vi "Text control 2 v6.2.vi"() -> ()   [LabVIEW 2016]
panel:
  in  "Tab Control":enum32{"Main", "Other parameters"}(tab)
  out "Line running":i32
  out "Total lines":i32
  out "Path":path=path "C:/users/rlp38/09Apr2009LTtesting/test2.txt"
  out "I vs Vg":cluster{"Y data in":dbl[], "X data in":dbl[]}[](graph)
  out "Is max":dbl format="%.2e"
  out "Id max":dbl format="%.2e"
  out "Ig max":dbl format="%.2e"
  out "Imax vs time":cluster{"Y data in":dbl[], "X data in":dbl[]}[](graph)
  out "Imin vs time":cluster{"Y data in":dbl[], "X data in":dbl[]}[](graph)
  out "I vs Vd":cluster{"Y data in":dbl[], "X data in":dbl[]}[](graph)
  in  "Script":string="#pulsedstressV d 0.03 20 0 0.5 0.0827 5\n#\n#itime m\n#gaterangemode a\n#drainrangemode a\n#pulsed on 0.05 0 0.02\n#transfer d -10 40 1 5 40 35\n#transfer d -10 40 1 5 40 35\n#transfer d -10 40 1 5 40 35\n#output d 0 40 20 0 40 1\n#\n#\n#sample 1 0.008 221 6 0.003\n#samplei 400e-6 200 6 0.002 0.1\n#vsu2pulse -10 4\n#\n#stressV 0.016 0.03 2e-4 0.1e-3 11\n#stressI 220e-7 0.08 15\n#transfer s -1 1 0.5 -0.005 0.005 0.005\n#output s 0 0 0 -0.008 0.008 0.002"
  out "Command running:":string
  out "Serial port data":string
  out "Elapsed Time":dbl caption="Elapsed Time (s)"
  in  "Time Units":u16(ring)=1 items=["Seconds", "Minutes", "Hours"]
  in  "Time Offset":dbl caption="Set Start Time (s)"
  in  "Reset":bool
  in  "Auto Reset":bool
  in  "integration time":u32(slide) max=2 step=1 scale=0.0..2.0
  out "Is on":dbl format="%.2e"
  out "Id on":dbl format="%.2e"
  out "Ig on":dbl format="%.2e"
  out "Ion vs time":cluster{"Y data in":dbl[], "X data in":dbl[]}[](graph)
  out "Ioff vs time":cluster{"Y data in":dbl[], "X data in":dbl[]}[](graph)
  out "Ig min":dbl format="%.2e"
  out "Id min":dbl format="%.2e"
  out "Is min":dbl format="%.2e"
  out "Is off":dbl format="%.2e"
  out "Id off":dbl format="%.2e"
  out "Ig off":dbl format="%.2e"
  in  "Integration time (long)":dbl=0.32 min=0.04 max=2.0 step=0.02 format="%.2f"
  in  "Integration time (short)":dbl=0.0019 min=8e-05 max=0.0019 step=8e-05 format="%^.0e"
  in  "Drain: Compliance":dbl=0.001 format="%.8f"
  in  "Gate: Compliance":dbl=0.001 format="%.8f"
  in  "Interrupt scan":bool
  in  "Standby":T1
  in  "Full Reset":bool
  in  "SMU4":cluster{"on/off":bool, "Voltage":dbl} {"Voltage" min=-100.0 max=100.0 format="%.2f"}
  in  "Interrupt program":bool
  in  "Gate Range\nmode":u16(ring) items=["Auto", "Limited", "Fixed"]
  in  "Gate Range":u8(slide)=6 max=11 scale=0.0..11.0
  in  "Source/Drain\nRange mode":u16(ring) items=["Auto", "Limited", "Fixed"]
  in  "Source/Drain Range":u8(slide)=6 max=11 scale=0.0..11.0
  in  "Panel Controls":T2={"Emergency Stop"=refnum, "TransGraph Max"=1e-05, "Text/Graph (text=false)"=TRUE} {"TransGraph Max" format="%.2e"}
  in  "Panel Controls 2":T3={"Emergency Stop"=refnum, "TransGraph Max"=1e-05, "Text/Graph (text=false)"=TRUE, "TransGraph Min"=1e-11} {"TransGraph Min" format="%.2e"; "TransGraph Max" format="%.2e"}
  out "error out":errorcluster
  in  "Delay before read (ms)":u32=1000
  in  "byte count":u32=64
  in  "Serial End Mode for Reads":u16(ring)=2 items=["None", "LastBit", "TermChar"]
  in  "Timeout (ms)":u32=10000
  in  "Enable Termination\nChar (T)":bool=TRUE
  in  "Termination char\n(0xA = '\\n' = LF)\n(0xD = '\\r' = CR)":u8=13 format="%.0x"
  in  "flow control":u16(ring) items=["None"=0, "XON/XOFF"=1, "RTS/CTS"=2, "DTR/DSR"=4]
  in  "stop bits":u16(ring)=10 items=["1.0"=10, "1.5"=15, "2.0"=20]
  in  "parity":u16(ring) items=["None", "Odd", "Even", "Mark", "Space"]
  in  "data bits":u16=8 min=5 max=8 step=1
  in  "VISA resource name":refnum<visa-resource-name>="COM6"
  in  "baud rate":u32=9600
  out "Timings Indicator":T4
  in  "Timings (overwritten by the Front Panel)":T5={"integration time"=0, "Short/Long integration time"=0.00064, "hold time (sec)"=0.0, "delay time (sec)"=0.0, "Step Time (0 disables)"=0.0, "sweep method"=0, "Pulse period"=0.005, "Base voltage"=0.0, "Pulse width"=0.0005} {"Pulse width" min=0.0005 max=0.1 step=0.0001 format="%.4f"; "Base voltage" format="%^.4e"; "Pulse period" min=0.005 max=1.0 step=0.0001 format="%.4f"; "sweep method" items=["Continuous", "Pulsed"]; "Step Time (0 disables)" format="%.2f"; "delay time (sec)" format="%.4f"; "hold time (sec)" format="%.4f"; "Short/Long integration time" format="%^.0e"; "integration time" scale=0.0..2.0}
  in  "Gate":T6={"Gate Start"=0.0, "Gate Stop"=2.0, "Gate Step (linear only)"=1.0, "Gate Compliance"=0.0001, "Gate PComp"=0.0, "Range mode"=0, "Range"=6} {"Range" max=11 scale=0.0..11.0; "Range mode" items=["Auto", "Limited", "Fixed"]; "Gate PComp" format="%^.2e"; "Gate Compliance" format="%^.2e"; "Gate Step (linear only)" format="%^.4e"; "Gate Stop" format="%^.4e"; "Gate Start" format="%^.4e"}
  in  "Drain 2":T7={"Drain Start"=0.0, "Drain Stop"=2.0, "Drain Compliance"=0.0001, "Drain Step"=1.0, "Drain PComp"=0.0, "Range mode"=0, "Range"=6} {"Range" max=11 scale=0.0..11.0; "Range mode" items=["Auto", "Limited", "Fixed"]; "Drain PComp" format="%^.2e"; "Drain Step" format="%^.4e"; "Drain Compliance" format="%^.2e"; "Drain Stop" format="%^.4e"; "Drain Start" format="%^.4e"}
  # "Time"
  # "Syntax:\nitime [s|m|l] time(sec): [s|m|l] determines the integration time setting (small|medium|long) and time sets the value.\nNOTE: The value of the integration time has to be within the range allowed by its category (s|m|l), otherwise, the closest value will be used. (e.g. if the category is set to short but the time value is very long, the actual value used will be the maximum short integration time.\nIntegration times:\n    Short: Default: 640 us. Range: 8E-5 - 1.92E-3 seconds.\n    Medium: Fixed at 1 NPL cycle (0.02 seconds).\n    Long: Default: 16 NPL cycles (0.32 seconds). Range: 2-100 NPL cycles (0.04 seconds - 2 seconds).\ngaterangemode [a|l|f]\ndrainrangemode [a|l|f]\npulsed [on|off] PulsePeriod(sec) PulseBaseVoltage PulseONWidth(sec)\nstandby [on l off]\nwait NumMilliseconds\nwait-min NumMinutes\n# texthere = comment\ntransfer [s|d] VgStart VgStop VgStep VdStart VdStop VdStep\noutput [s|d] VgStart VgStop VgStep VdStart VdStop VdStep\nsample Vg Vd NumSamples Time(s) SampleInterval(s)\nsamplei Idg NumSamples Time(s) SampleInterval(s) VDGcompliance\n100 samples is approximately 13 seconds with medium integration\n# if in doubt use SampleInterval(s) = 0.004\nstressV VG VD IGcompliance IDcompliance Duration(sec)\nstressI IDG VDGcompliance Duration(sec)\nvsu2pulse Bias Duration(s)\npulsedstressV [s|d] VEstop VgON VgOFF Period(s) PulseONwidth(s) Vd\nsample-fpp Vg Vd NumSamples Time\nresample-fpp Vg Vd\ntransfer-fpp [s|d] VgStart VgStop VgStep VdStart VdStop VdStep\noutput-fpp [s|d] VgStart VgStop VgStep VdStart VdStop VdStep\nserial SerialPortCommand"
  # "1\n2\n3\n4\n5\n6\n7\n8\n9\n10\n11\n12\n13\n14\n15\n16\n17\n18\n19\n20"
  # "Serial port settings"
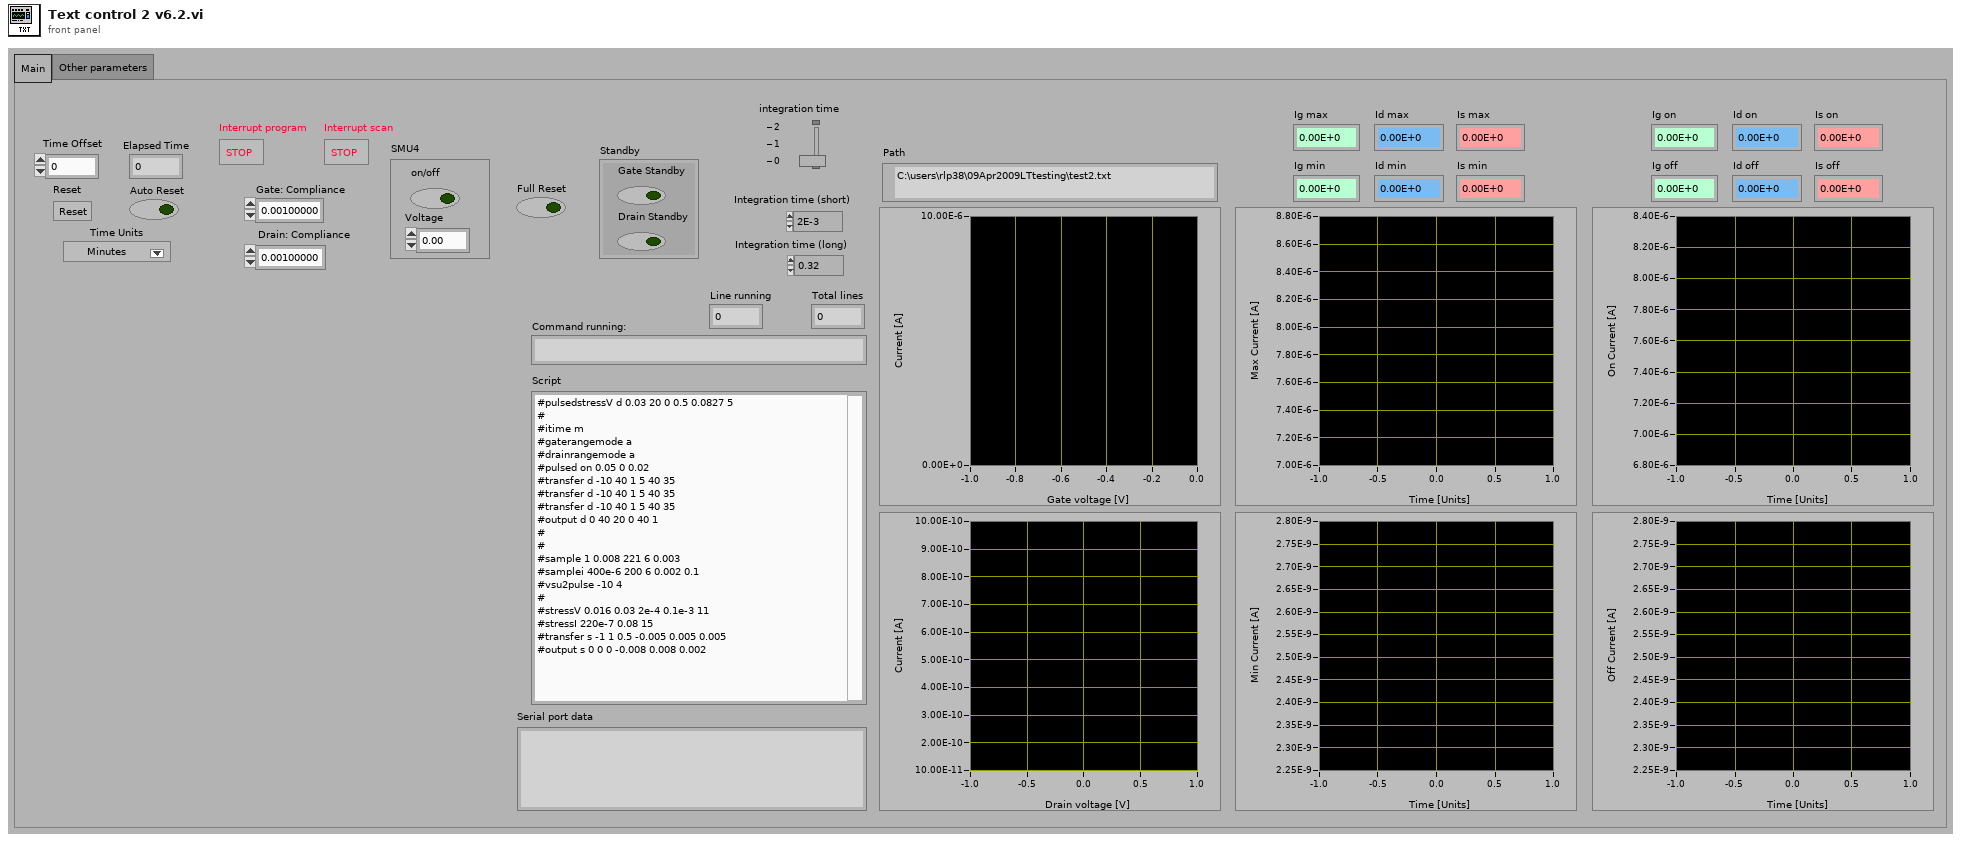
[diagram p1: front panel]
types:
  T1 = cluster{"Gate Standby":bool, "Drain Standby":bool}
  T2 = cluster{"Emergency Stop":refnum<vi>, "TransGraph Max":dbl, "Text/Graph (text=false)":bool}
  T3 = cluster{"Emergency Stop":refnum<vi>, "TransGraph Max":dbl, "Text/Graph (text=false)":bool, "TransGraph Min":dbl}
  T4 = cluster{"integration time (0:s, 1:m, 2:l)":u32, "Short/Long integration time":dbl, "hold time (sec)":dbl, "delay time (sec)":dbl, "Step Time (0 disables)":dbl, "sweep method":u16, "Pulse period":dbl, "Base voltage":dbl, "Pulse width":dbl}
  T5 = cluster{"integration time":u32, "Short/Long integration time":dbl, "hold time (sec)":dbl, "delay time (sec)":dbl, "Step Time (0 disables)":dbl, "sweep method":u16, "Pulse period":dbl, "Base voltage":dbl, "Pulse width":dbl}
  T6 = cluster{"Gate Start":dbl, "Gate Stop":dbl, "Gate Step (linear only)":dbl, "Gate Compliance":dbl, "Gate PComp":dbl, "Range mode":u16, "Range":u8}
  T7 = cluster{"Drain Start":dbl, "Drain Stop":dbl, "Drain Compliance":dbl, "Drain Step":dbl, "Drain PComp":dbl, "Range mode":u16, "Range":u8}
  T8 = enum16{"open", "replace", "create", "open or create", "replace or create", "replace or create with confirmation"}
  T9 = cluster{"V2 Start":dbl, "V2 Step":dbl, "Number of points":i32}
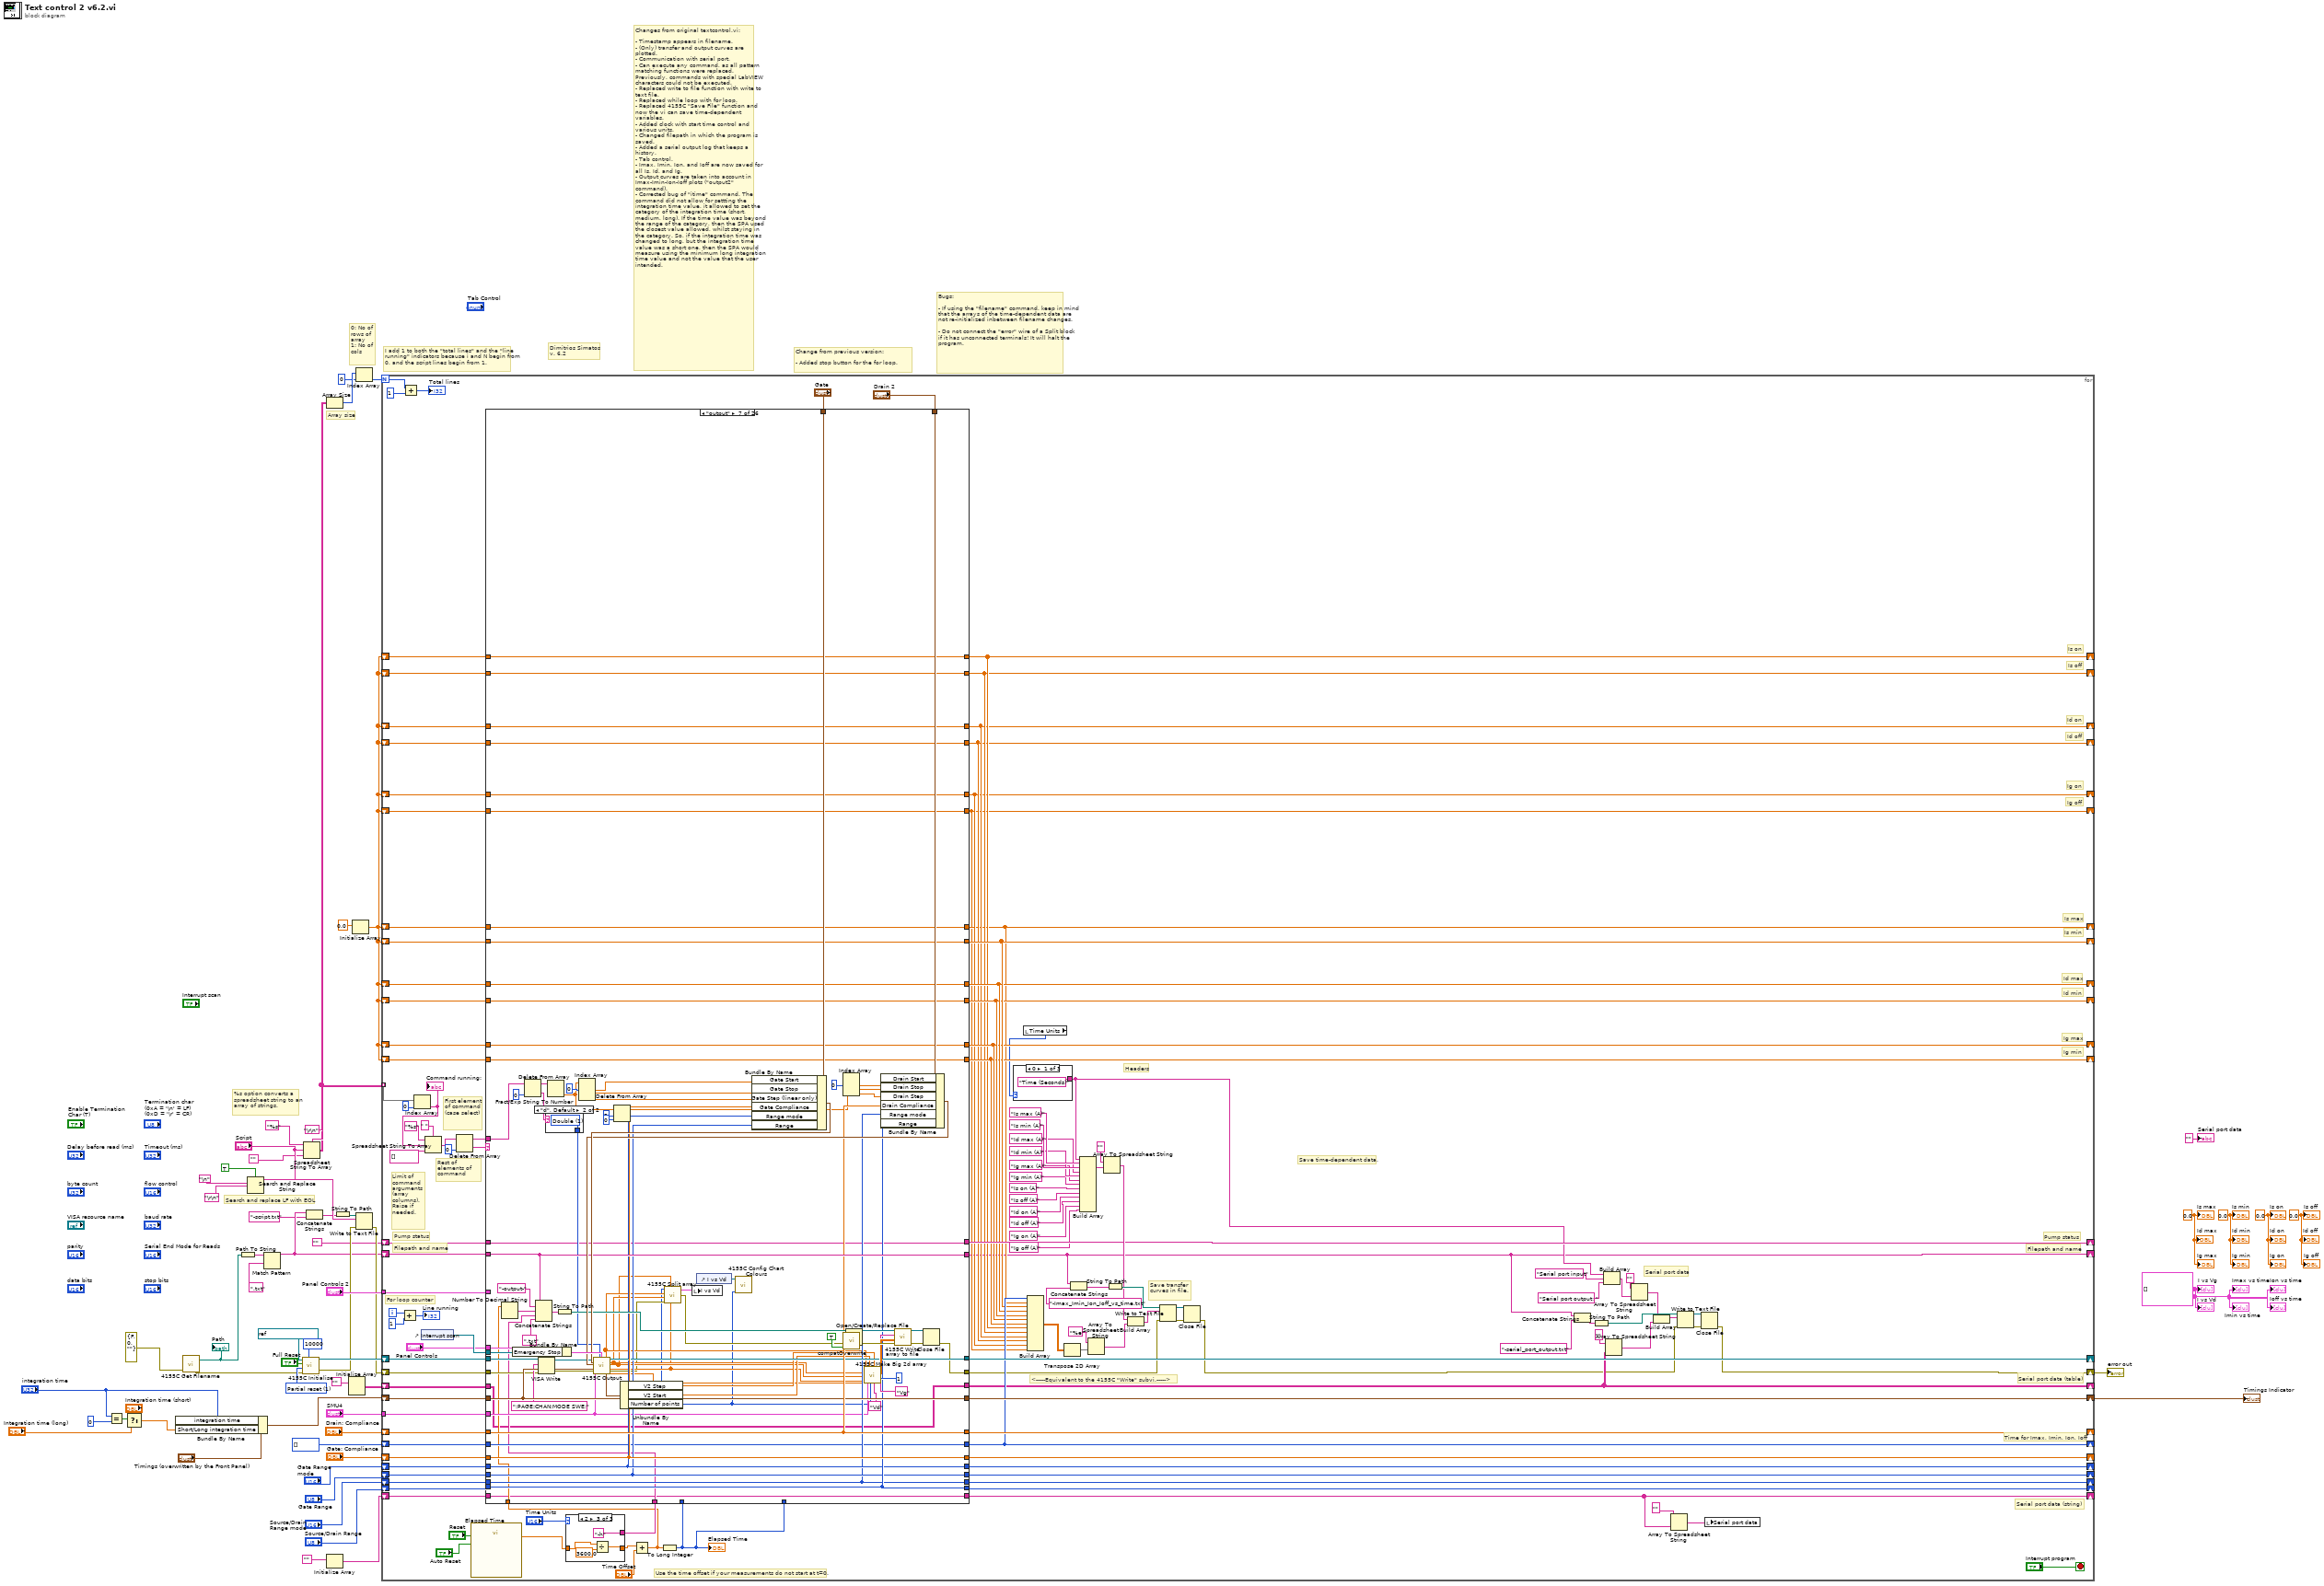
[diagram p0: block diagram]
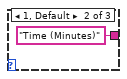
[diagram p2: hidden frame]
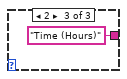
[diagram p3: hidden frame]
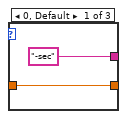
[diagram p4: hidden frame]
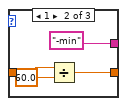
[diagram p5: hidden frame]
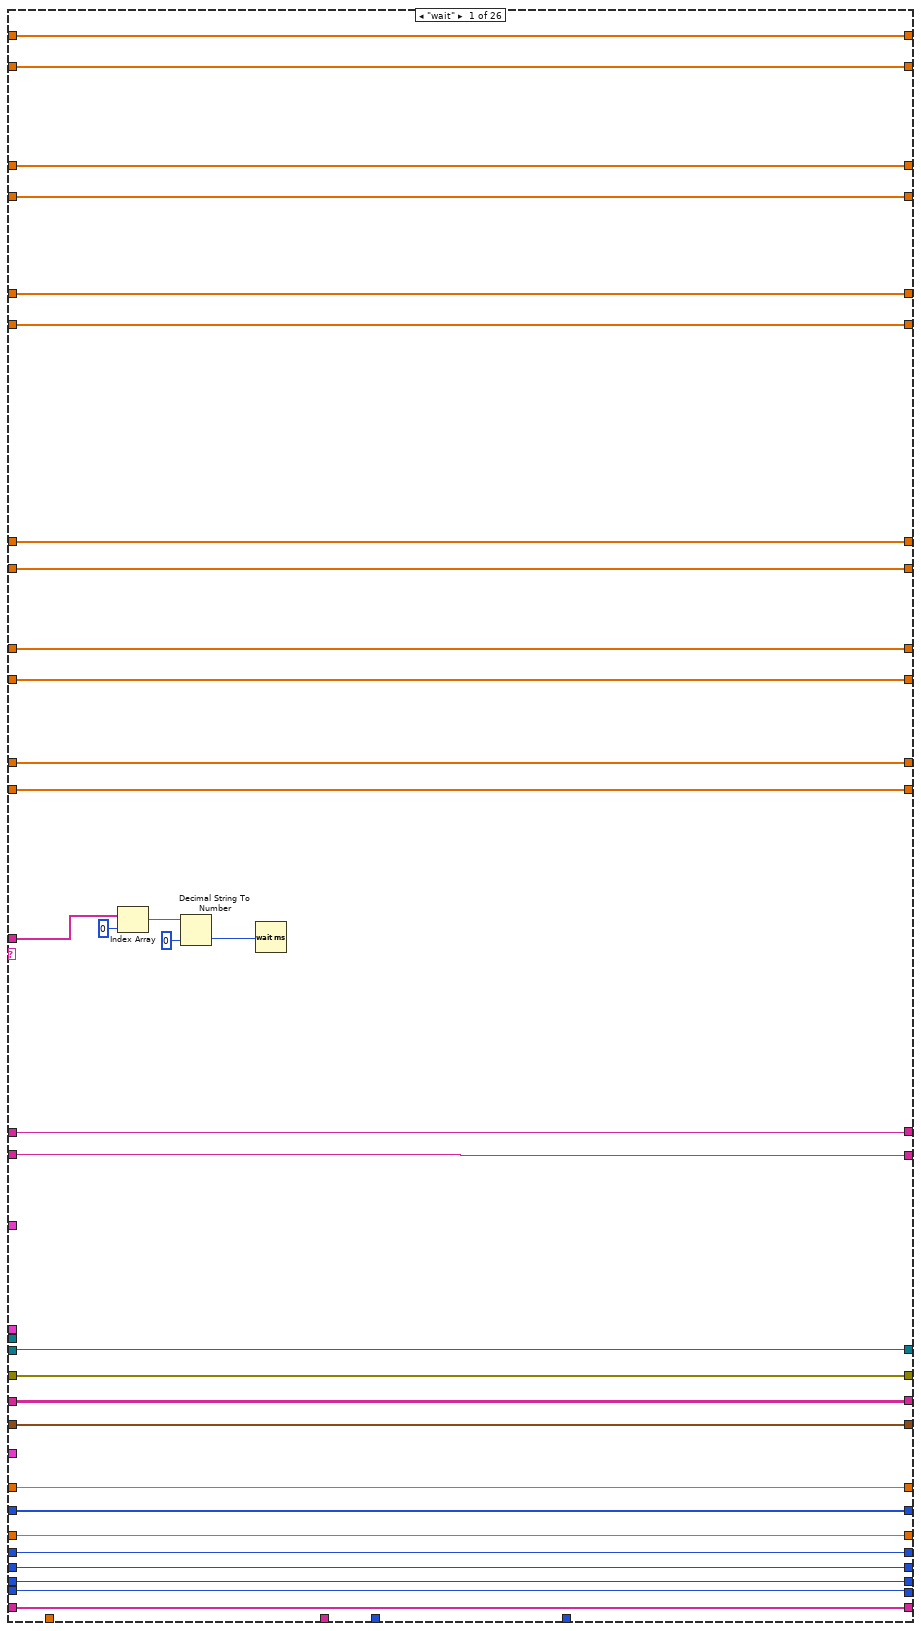
[diagram p6: hidden frame]
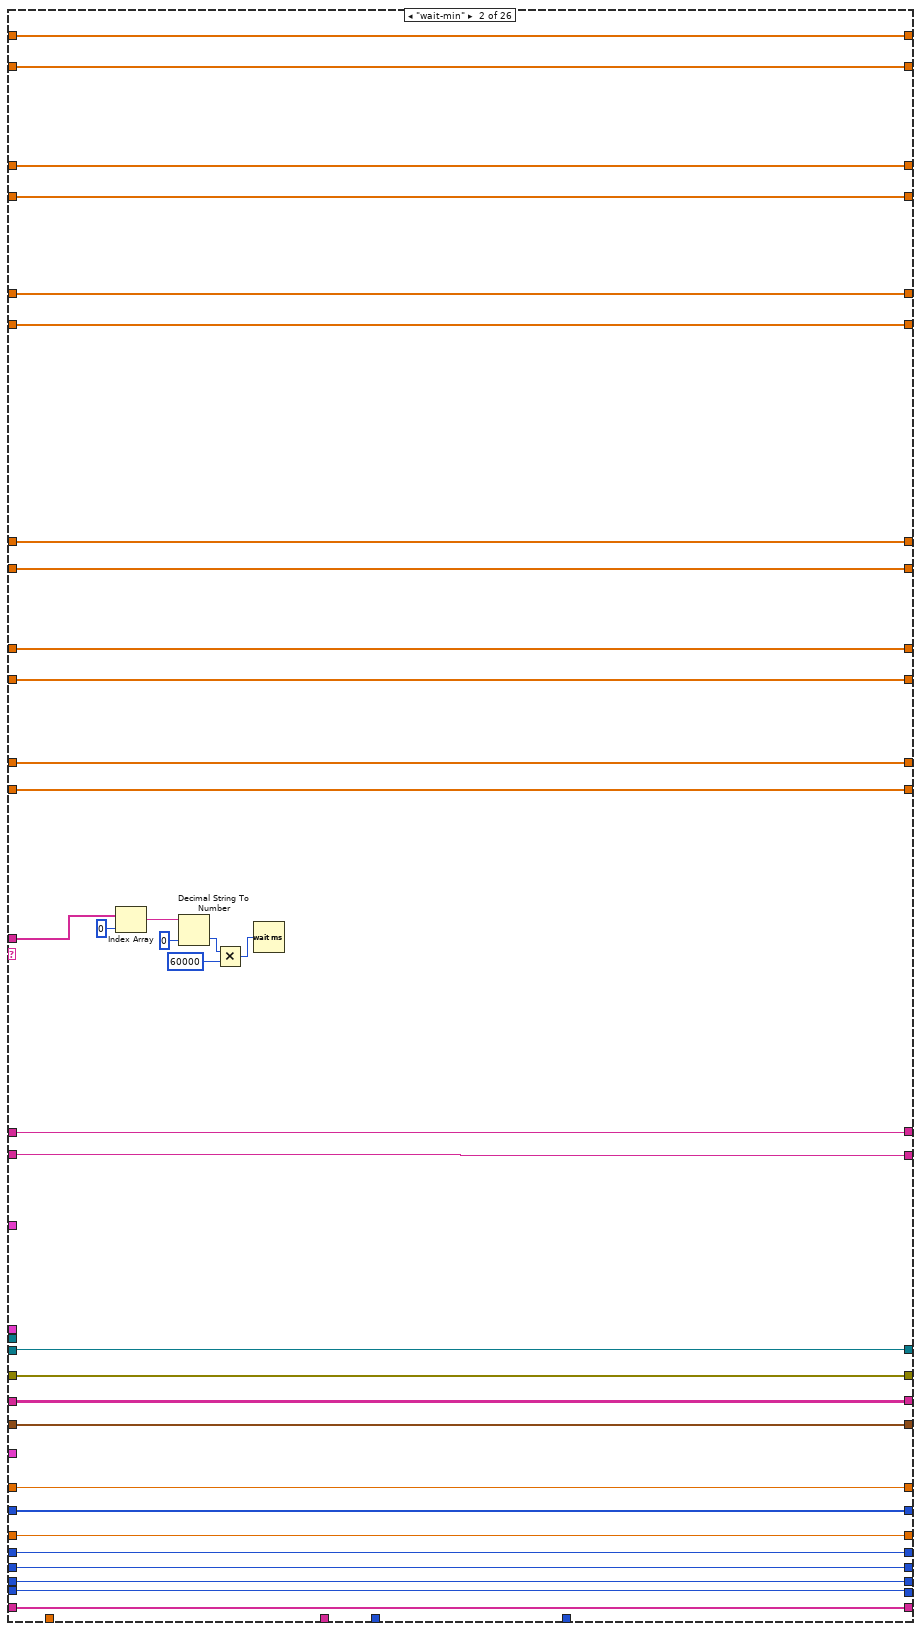
[diagram p7: hidden frame]
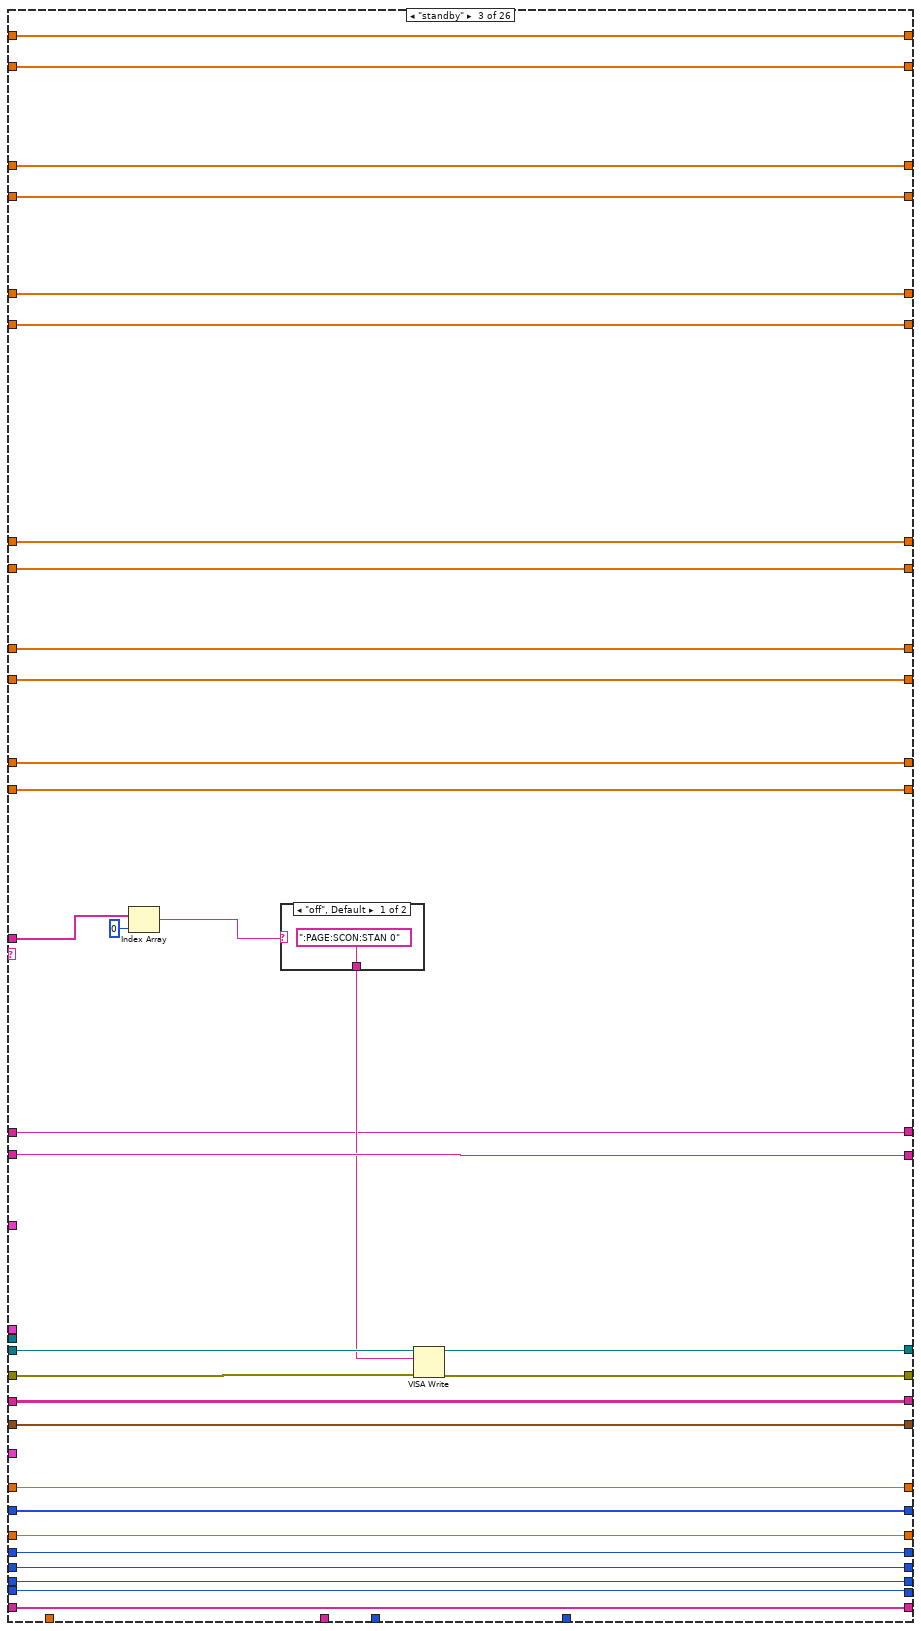
[diagram p8: hidden frame]
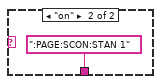
[diagram p9: hidden frame]
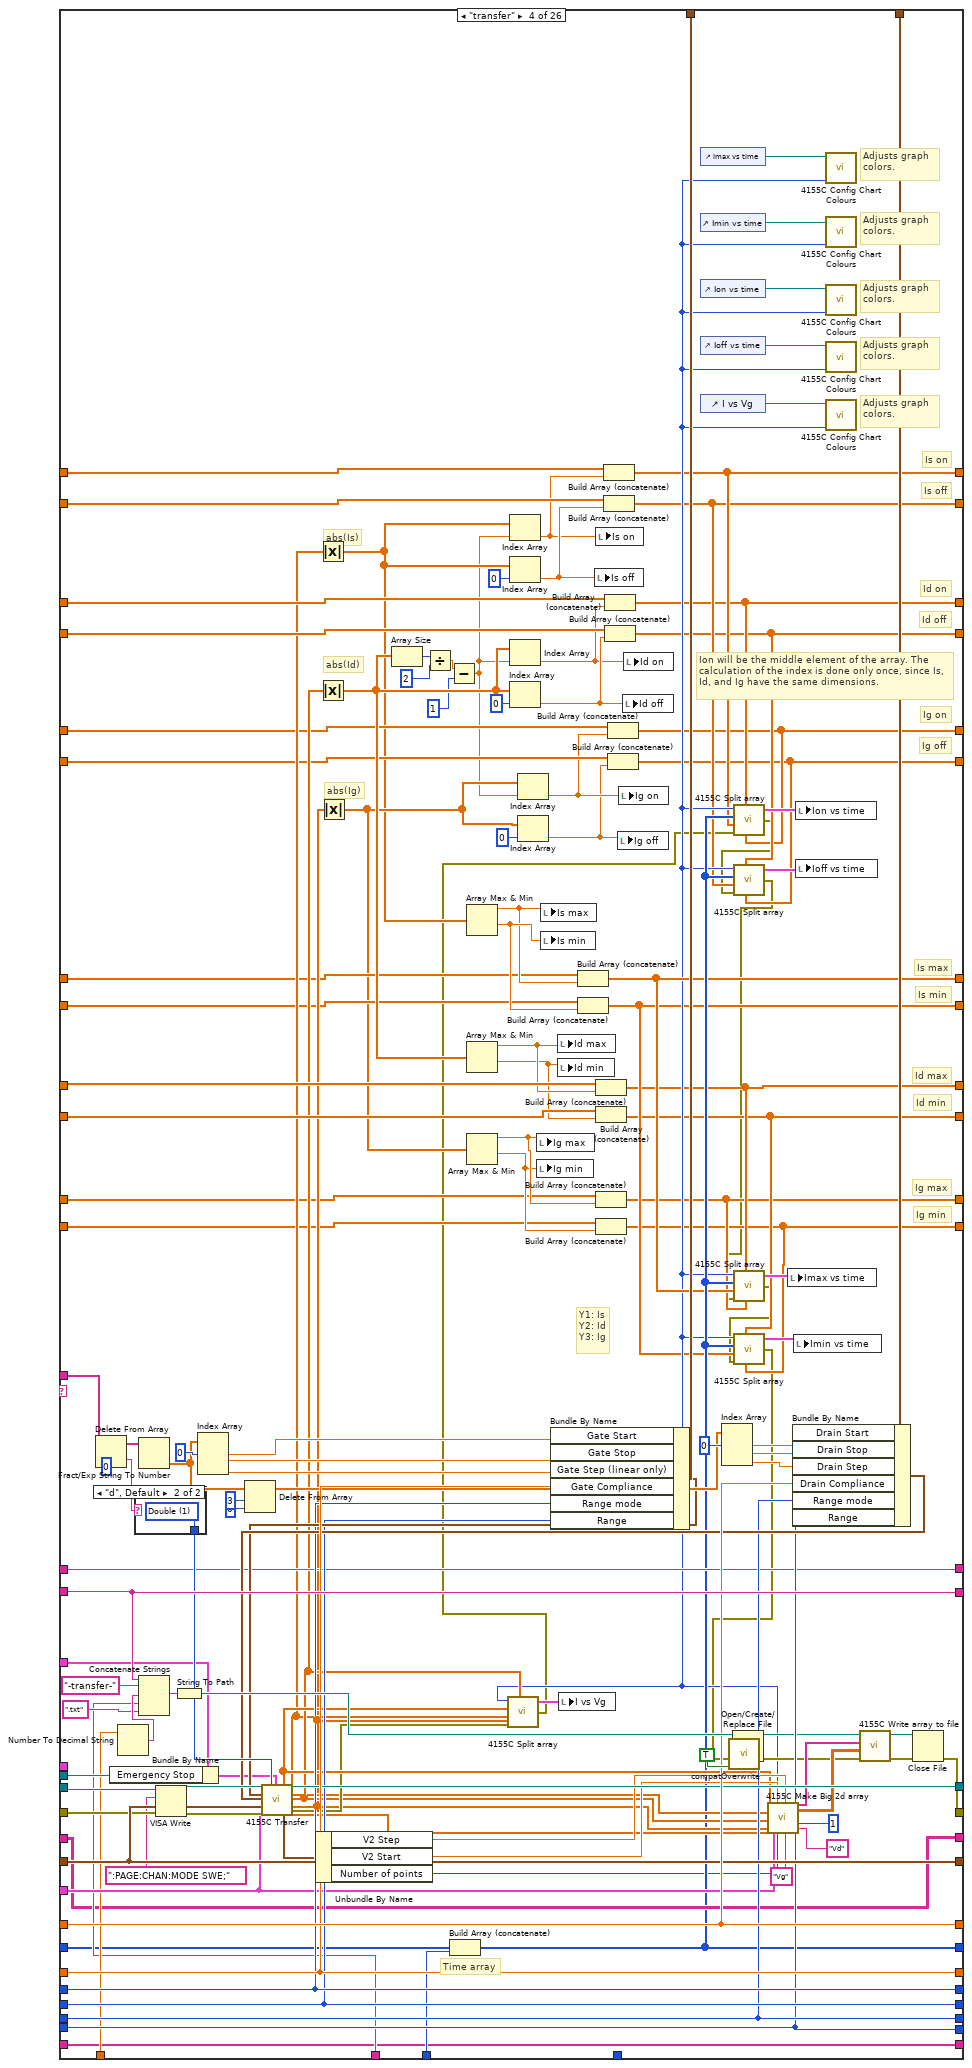
[diagram p10: hidden frame]
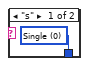
[diagram p11: hidden frame]
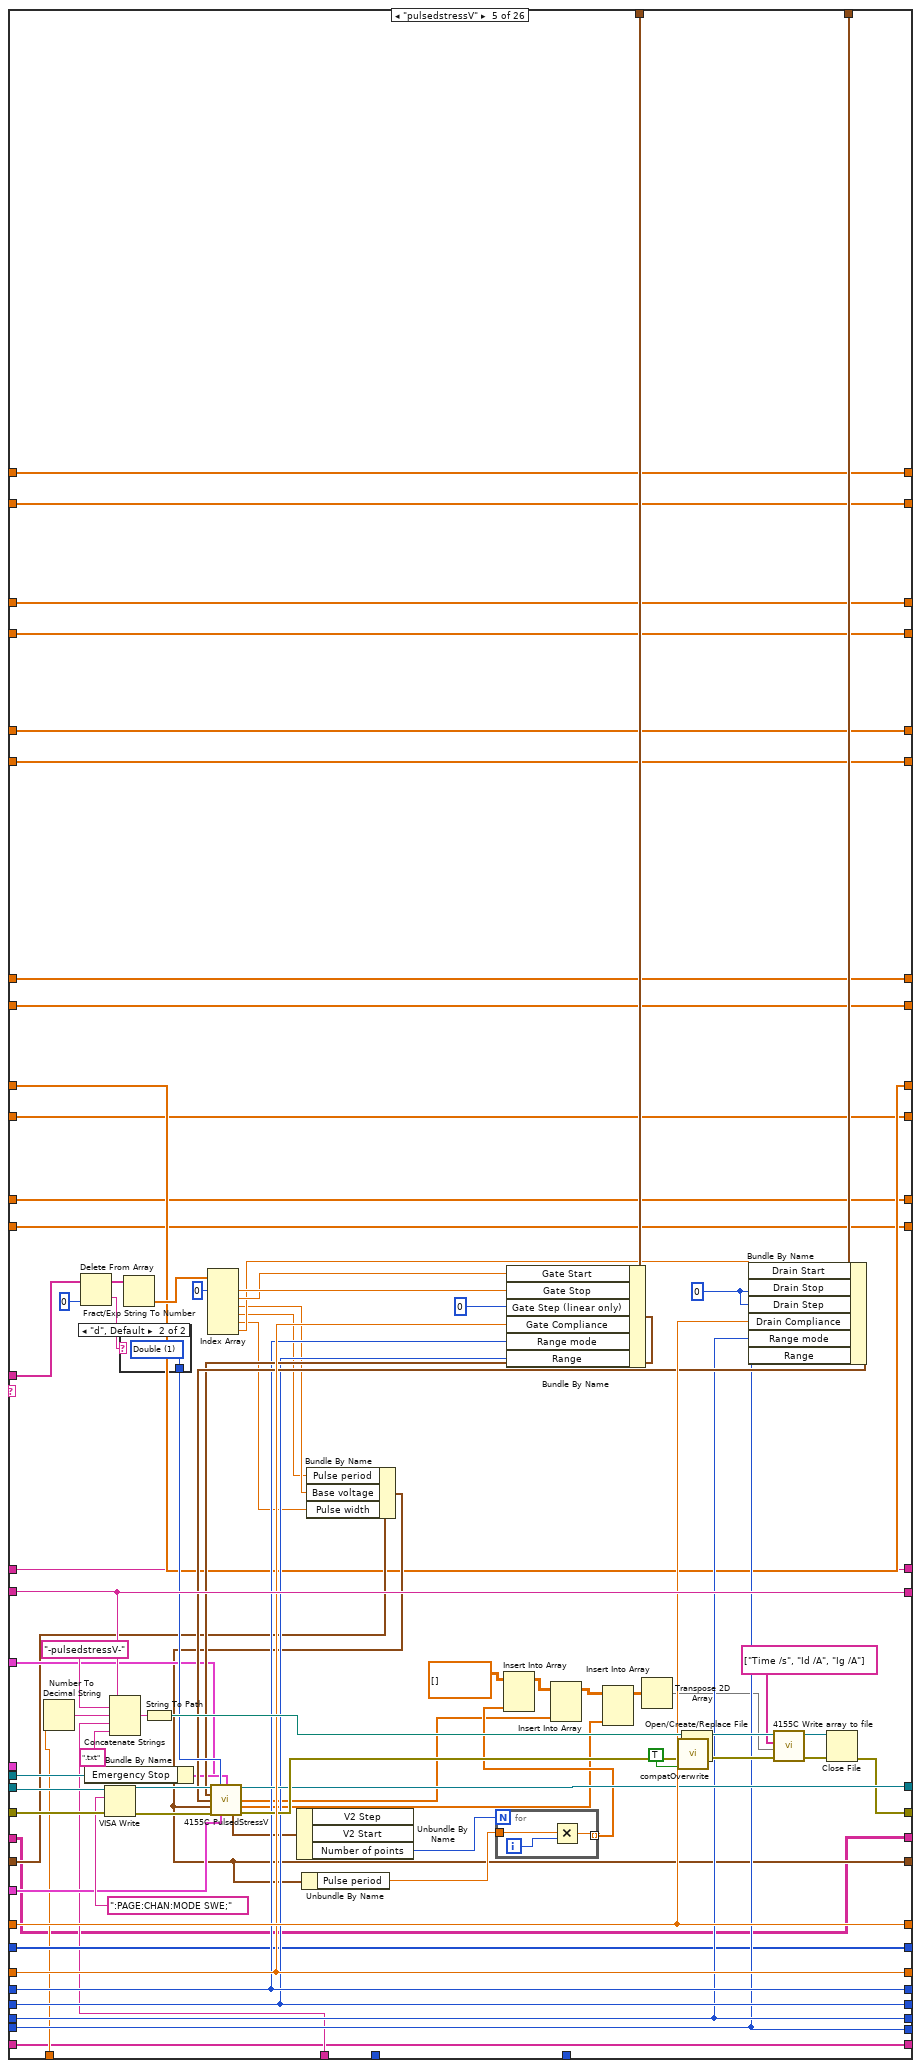
[diagram p12: hidden frame]
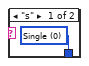
[diagram p13: hidden frame]
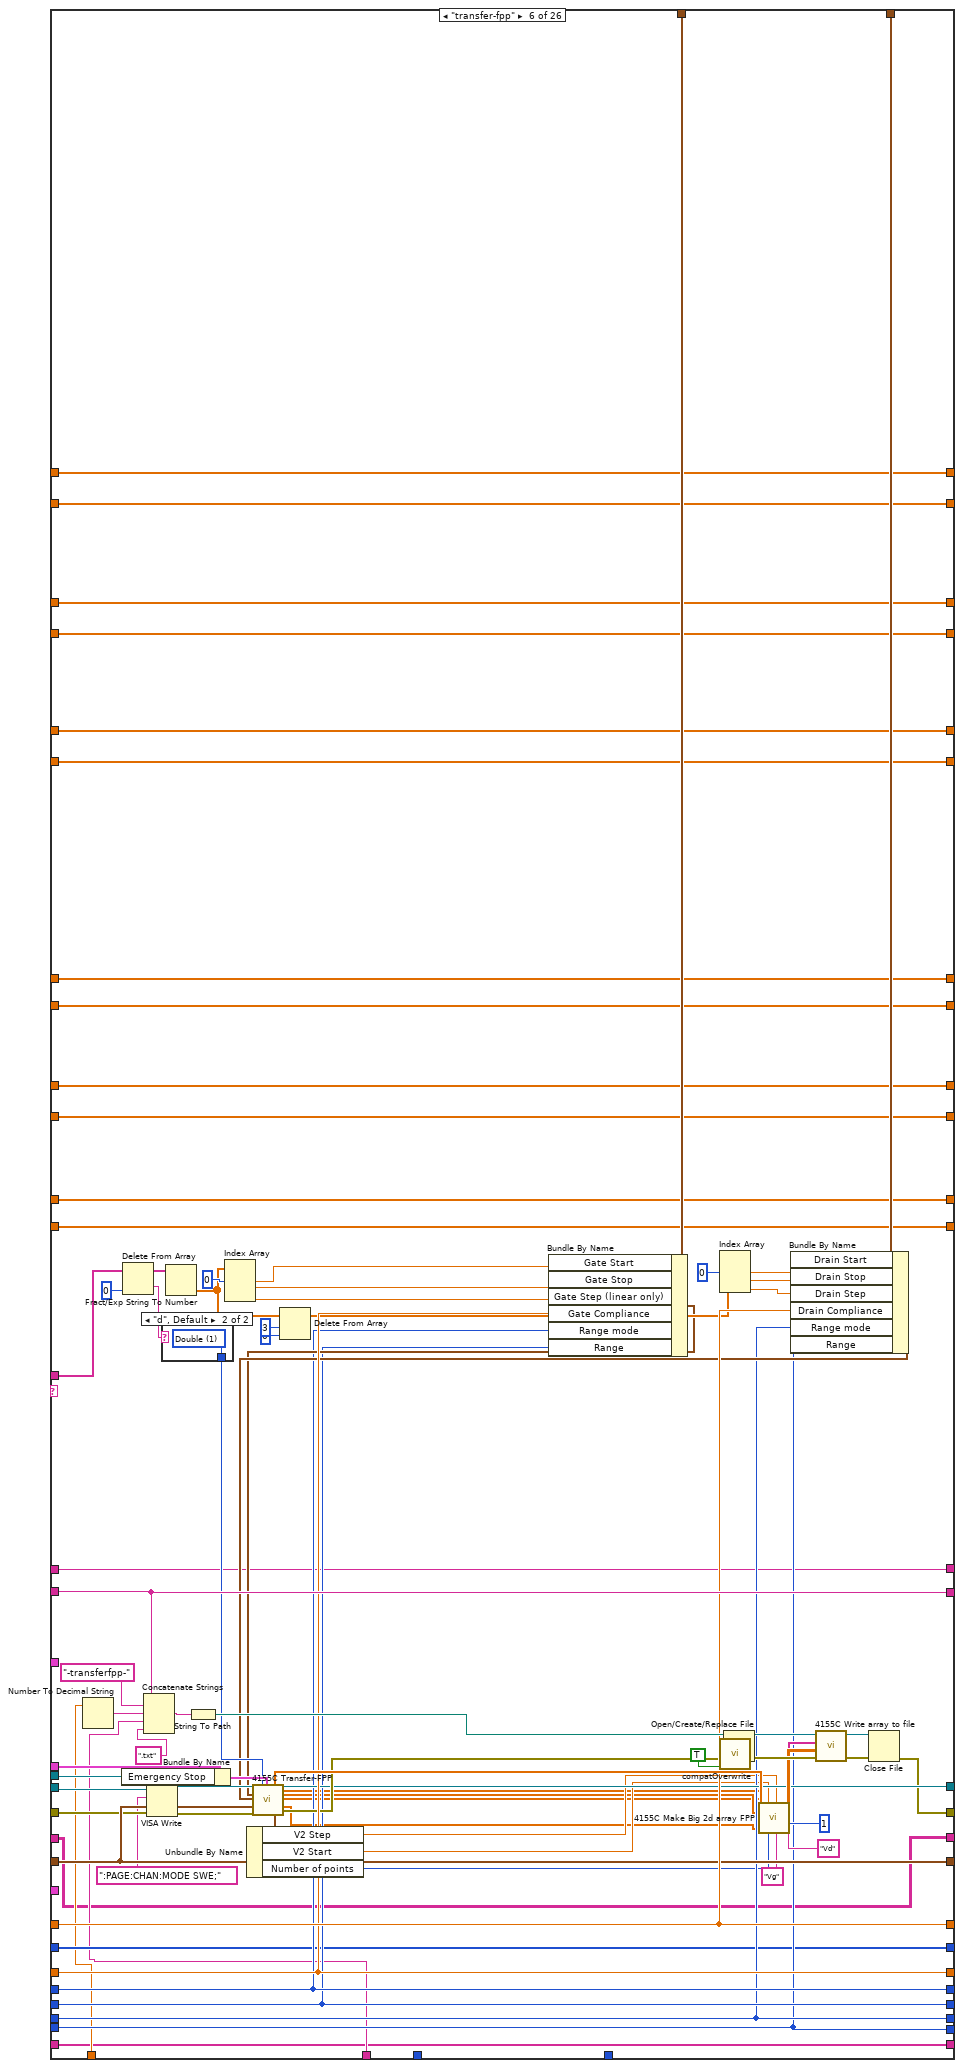
[diagram p14: hidden frame]
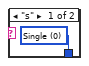
[diagram p15: hidden frame]
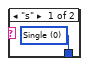
[diagram p16: hidden frame]
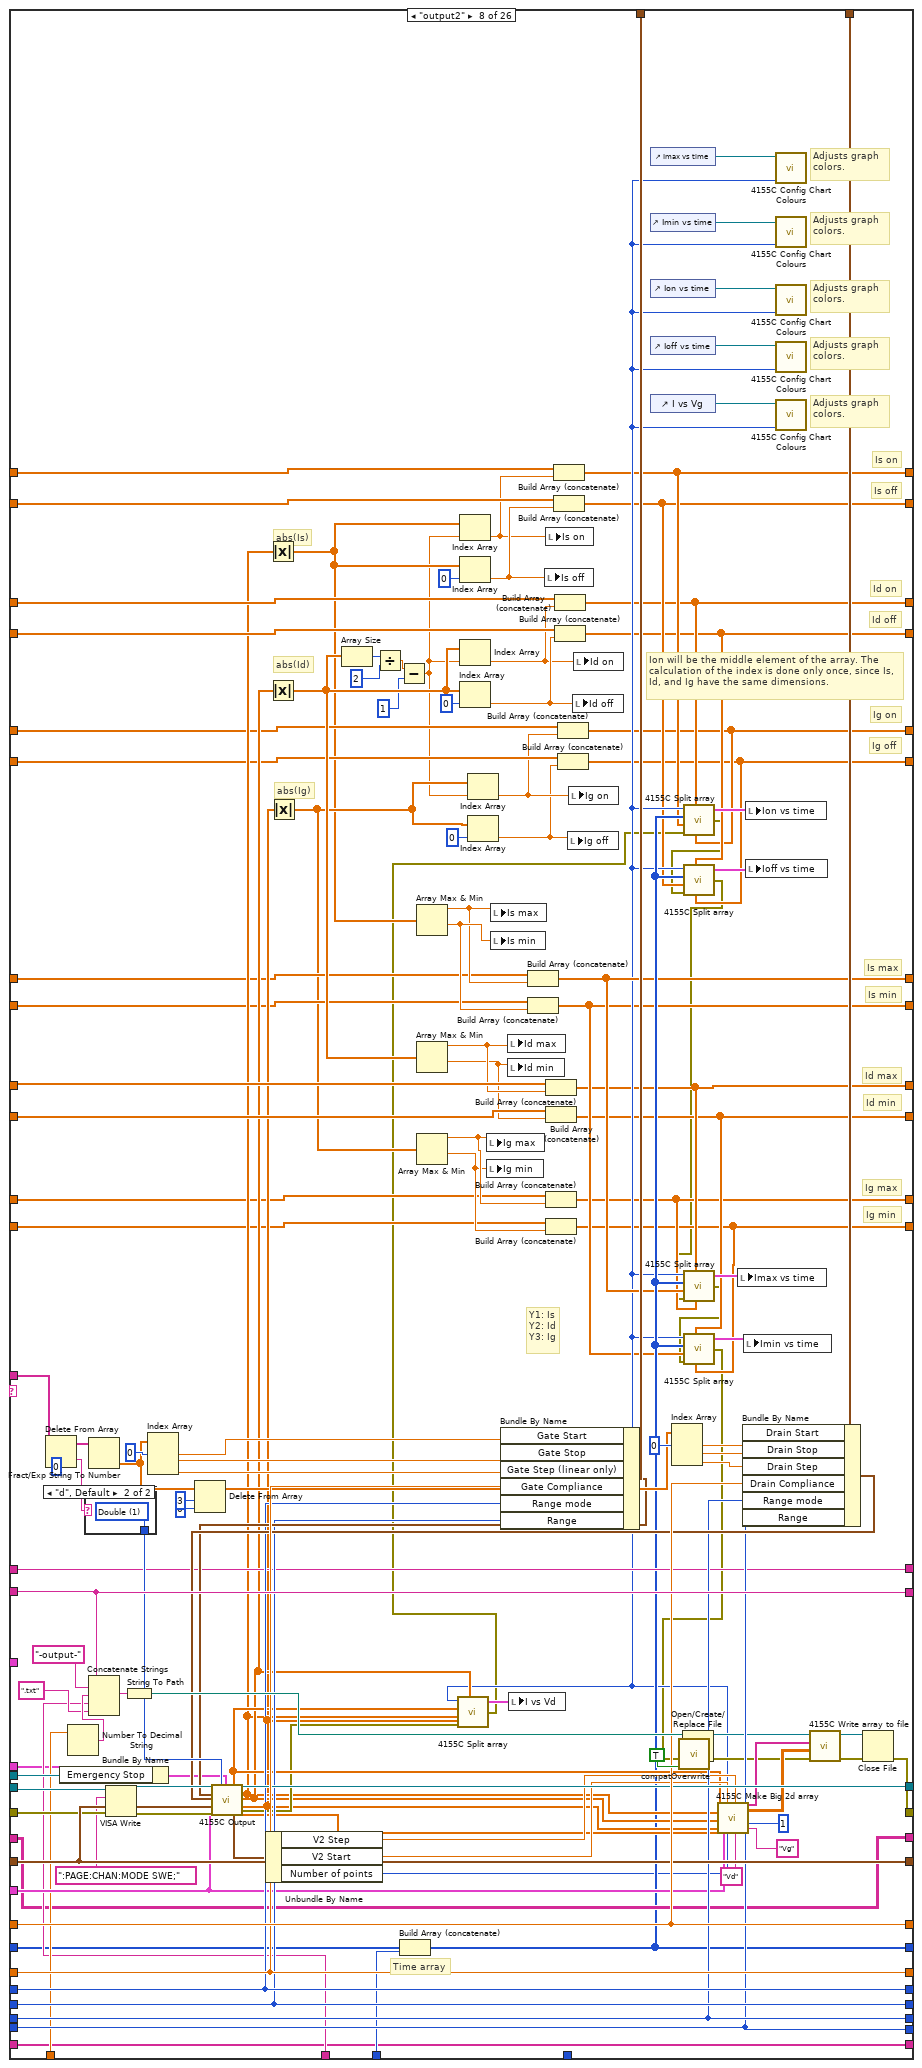
[diagram p17: hidden frame]
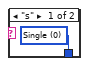
[diagram p18: hidden frame]
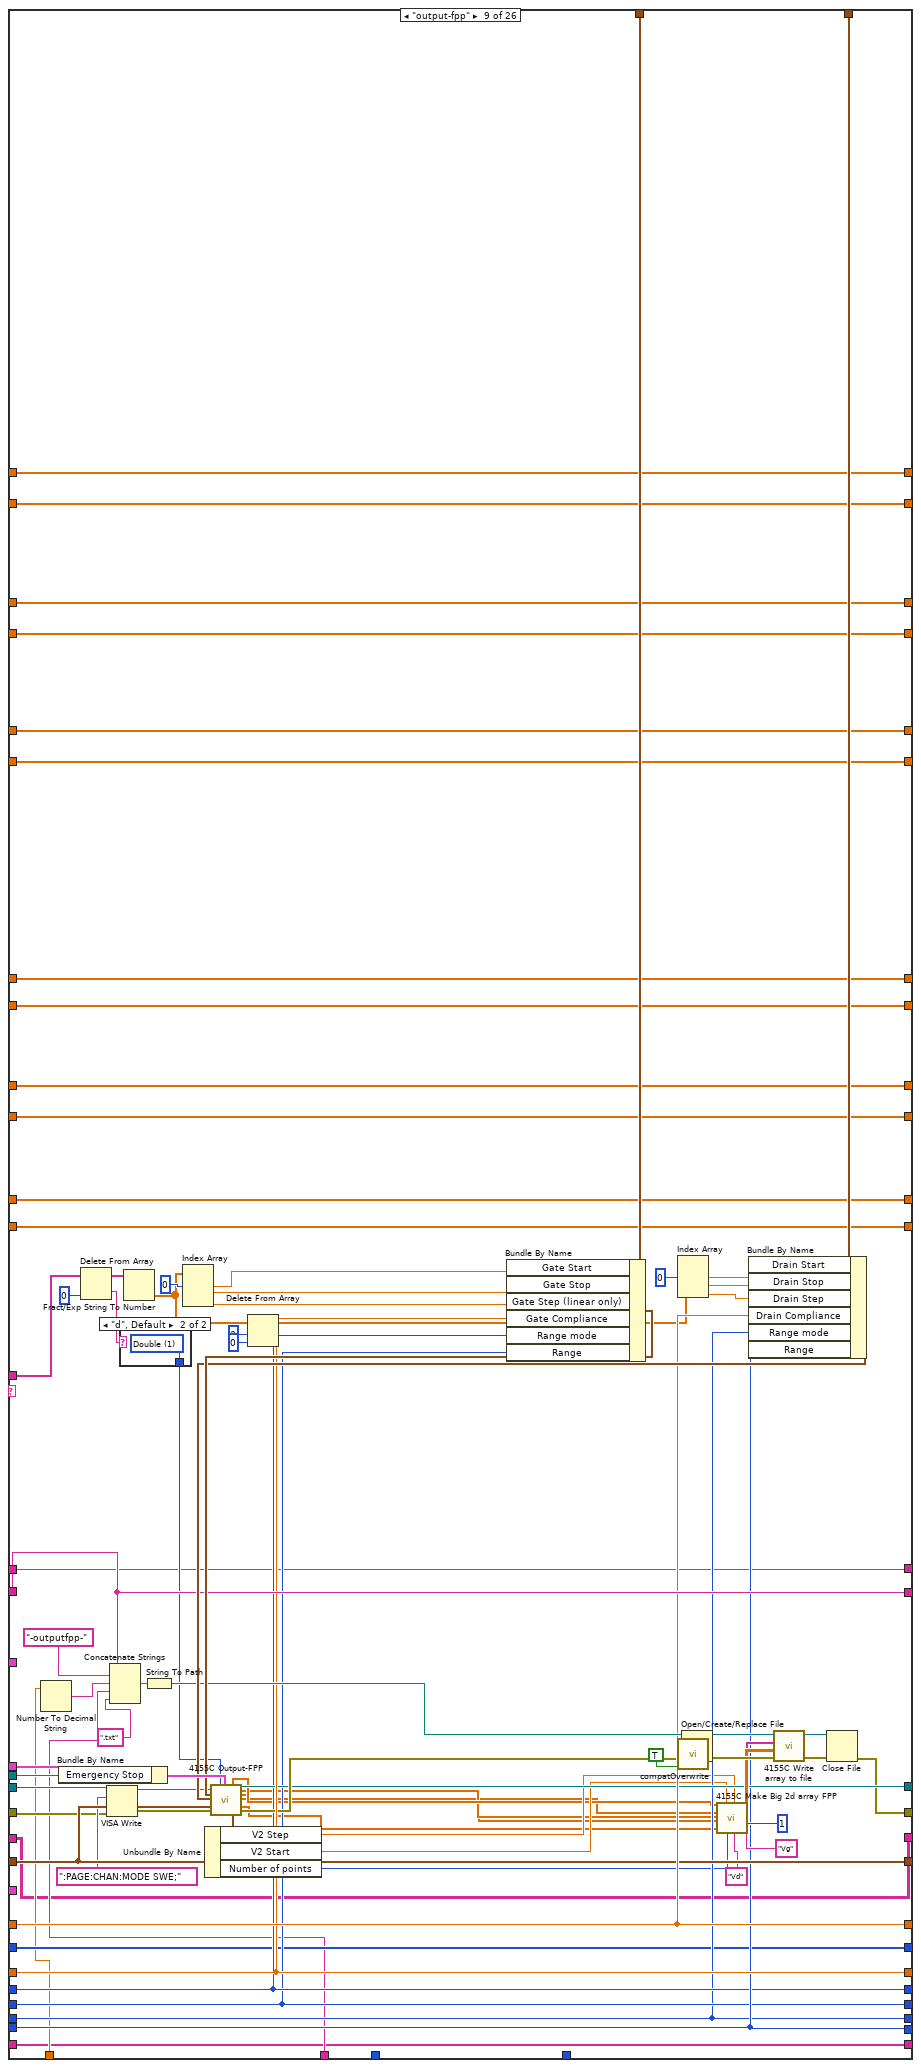
[diagram p19: hidden frame]
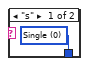
[diagram p20: hidden frame]
diagram:
  w2 = cluster{"Y data in":dbl[], "X data in":dbl[]}[] [] ("I vs Vg")
  w3 = 0.0 ("Is off")
  w4 = 0.0 ("Is on")
  w5 = 0.0 ("Is min")
  w6 = 0.0 ("Is max")
  w55 = u16 1 items=["Reset All", "Partial reset"] ("Type of reset")
  # "Change from previous version:\n\n- Added stop button for the for loop."
  # "I add 1 to both the \"total lines\" and the \"line running\" indicators because i and N begin from 0, and the script lines begin from 1."
  # "Bugs:\n\n- If using the \"filename\" command, keep in mind that the arrays of the time-dependent data are not re-initialized inbetween filename changes. \n\n- Do not connect the \"error\" wire of a Split block if it has unconnected terminals! It will halt the program."
  # "Array size"
  # "%s option converts a spreadsheet string to an array of strings."
  # "0: No of rows of array\n1: No of cols"
  # "Dimitrios Simatos\nv. 6.2"
  # "Changes from original textcontrol.vi:\n\n- Timestamp appears in filename.\n- (Only) transfer and output curves are plotted.\n- Communication with serial port.\n- Can execute any command, as all pattern matching functions were replaced. Previously, commands with special LabVIEW characters could not be executed.\n- Replaced write to file function with write to text file.\n- Replaced while loop with for loop.\n- Replaced 4155C \"Save File\" function and now the vi can save time-dependent variables.\n- Added clock with start time control and various units.\n- Changed filepath in which the program is saved.\n- Added a serial output log that keeps a history.\n- Tab control.\n- Imax, Imin, Ion, and Ioff are now saved for all Is, Id, and Ig.\n- Output curves are taken into account in Imax-Imin-Ion-Ioff plots (\"output2\" command).\n- Corrected bug of \"itime\" command. The command did not allow for settting the integration time value, it allowed to set the category of the integration time (short, medium, long). If the time value was beyond the range of the category, then the SPA used the closest value allowed, whilst staying in the category. So, if the integration time was changed to long, but the integration time value was a short one, then the SPA would measure using the minimum long integration time value and not the value that the user intended."
  # "Search and replace LF with EOL"
  n1 = Equal?(x="integration time", y=u32 0) -> (x = y?=w56:bool)
  n2 = Select(t="Integration time (short)", s=w56, f="Integration time (long)") -> (s? t:f=w11:dbl)
  n3 = Bundle By Name(cluster="Timings (overwritten by the Front Panel)", "integration time"="integration time", "Short/Long integration time"=w11) -> (w48:T5)
  n4 = call "4155C Get Filename.vi"("error in (no error)"=errorcluster {"status"=FALSE, "code"=0, "source"=""}) -> ("error out"=w50:errorcluster, "path"=w25:path)  [unwired: 2 in, 1 out]
  "Path" <- w25
  n5 = Path To String(path=w25) -> (string=w26:string)
  n6 = Search and Replace String(replace all?=TRUE ("replace all? (F)"), input string="Script", search string="\n", replace string="\r\n") -> (result string=w38:string)  [unwired: 4 in, 3 out]
  n7 = Match Pattern(string=w26, regular expression=".txt") -> (before substring=w9:string)  [unwired: 1 in, 3 out]
  n8 = call "4155C Initialise.vi"("VISA resource name in"=refnum<visa-resource-name> "GPIB0::14::INSTR", "Reset"="Full Reset", "Type of reset"=w55, "error in (no error)"=w50, "VISA Timeout Value"=u32 10000) -> ("VISA Resource Name out"=w49:refnum<visa-resource-name>, "error out"=w21:errorcluster)
  n9 = Spreadsheet String To Array(delimiter (Tab)="\r\n", format string="%s", spreadsheet string="Script", array type (2D Dbl)="") -> (array=w29:string[][])
  n10 = Concatenate Strings(w9, "-script.txt" ("string")) -> (w10:string)
  n11 = Array Size(array=w29) -> (size(s)=w33:i32[])
  n12 = Initialize Array("") -> (w16:string[])  [unwired: 1 in]
  n13 = String To Path(string=w10) -> (path=w22:path)
  n14 = Initialize Array("") -> (w14:string[][])  [unwired: 2 in]
  n15 = Initialize Array(0.0 ("element")) -> (w18:dbl[])  [unwired: 1 in]
  n16 = Index Array(array=w33, index=0) -> (element=w31:i32)
  n17 = Write to Text File(file (use dialog)=w22, text=w38, error in=w21) -> (error out=w20:errorcluster)  [unwired: 1 in, 2 out]
  n18 = for {
    N: w31 -> [w130]
    tunnel: "SMU4" -> [w166]
    shift-left: "Source/Drain Range" -> [w171]
    shift-right: [w167] -> _
    shift-left: "Source/Drain\nRange mode" -> [w172]
    shift-right: [w168] -> _
    shift-left: "Gate Range" -> [w173]
    shift-right: [w169] -> _
    shift-left: "Gate Range\nmode" -> [w174]
    shift-right: [w170] -> _
    shift-left: "Gate: Compliance" -> [w183]
    shift-right: [w179] -> _
    shift-left: "Drain: Compliance" -> [w184]
    shift-right: [w180] -> _
    shift-left: w48 -> [w185]
    shift-right: [w181] -> w12
    shift-left: w20 -> [w186]
    shift-right: [w64] -> w24
    shift-left: w49 -> [w187]
    shift-right: [w182] -> _
    shift-left: w9 -> [w188]
    shift-right: [w67] -> _
    tunnel: "Panel Controls 2" -> [w165]
    shift-right: [w79] -> _
    shift-left: w18 -> [w164]
    shift-right: [w115] -> _
    shift-left: i32[] [] -> [w160]
    tunnel: w29 -> [w159] mode=indexing
    shift-right: [w78] -> _
    shift-left: w18 -> [w136]
    shift-right: [w109] -> _
    shift-left: w16 -> [w122]
    shift-right: [w117] -> _
    shift-left: "" -> [w116]
    shift-right: [w110] -> _
    shift-left: w14 -> [w112]
    shift-right: [w72] -> _
    shift-left: w18 -> [w100]
    shift-right: [w73] -> _
    shift-left: w18 -> [w99]
    shift-right: [w77] -> _
    shift-left: w18 -> [w88]
    shift-right: [w76] -> _
    shift-left: w18 -> [w87]
    shift-right: [w70] -> _
    shift-left: w18 -> [w86]
    shift-right: [w80] -> _
    shift-left: w18 -> [w85]
    shift-right: [w71] -> _
    shift-left: w18 -> [w84]
    shift-right: [w69] -> _
    shift-left: w18 -> [w83]
    shift-right: [w75] -> _
    shift-left: w18 -> [w82]
    shift-right: [w74] -> _
    shift-left: w18 -> [w81]
    i -> [w125]
    stop <- "Interrupt program" stop-if-true
    # "Is off"
    # "Is on"
    # "Ig off"
    # "Ig on"
    # "Is min"
    # "Is max"
    # "Ig min"
    # "Ig max"
    # "Id min"
    # "Id max"
    # "Id off"
    # "Id on"
    # "Pump status"
    # "Filepath and name"
    # "Pump status"
    # "Limit of command arguments (array columns). Raise if needed."
    # "Serial port data (string)"
    # "Serial port data (table)"
    # "Serial port data"
    # "For loop counter"
    # "<-----Equivalent to the 4155C \"Write\" subvi.----->"
    # "Headers"
    # "Save transfer curves in file."
    # "Filepath and name"
    # "Save time-dependent data."
    # "Use the time offset if your measurements do not start at t=0."
    # "Time for Imax, Imin, Ion, Ioff"
    # "Rest of elements of command"
    # "First element of command\n(case select)"
    n19 = Add(x=w125, y=1) -> (x+y=→"Line running":i32)
    n20 = Add(x=w130, y=1) -> (x+y=→"Total lines":i32)
    n21 = Index Array(array=w159, index=0 ("line index")) -> (element=w154:string)
    "Command running:" <- w154
    n22 = control-ref of="Interrupt scan"() -> (w178:refnum<vi>)
    n23 = Spreadsheet String To Array(delimiter (Tab)=" ", format string="%s", spreadsheet string=w154, array type (2D Dbl)=string[] []) -> (array=w152:string[])
    n24 = Delete From Array(array=w152, index=0) -> (deleted portion=w101:string, array with subset deleted=w151:string[])  [unwired: 1 in]
    n25 = call "Elapsed Time"("Reset"="Reset", "Auto Reset"="Auto Reset") -> ("Elapsed Time (s)"=w161:dbl)  [unwired: 10 in, 7 out]
    n26 = case shown="2" "Time Units" {
      tunnel: ["-sec" "-min" "-h"] -> w162
      tunnel: [w192 w196 w199] -> w132
      tunnel: w161 -> [w192 w195 w200]
      frame 0, Default {
      }
      frame 1 {
        n27 = Divide(x=w195, y=60.0) -> (x/y=w196:dbl)
      }
      frame 2 {
        n28 = Divide(x=w200, y=3600.0) -> (x/y=w199:dbl)
      }
    }
    n29 = Add(x=w132, y="Time Offset") -> (x+y=w131:dbl)
    n30 = To Long Integer(number=w131) -> (32bit integer=w114:i32)
    "Elapsed Time" <- w114
    n31 = case shown="\"output\"" w101 {
      tunnel: w151 -> [w232 w265 w297 w425 w448 w585 w675 w823 w896 w923 w993 w1034 w1073 w1108 w1136 _ _ w1282 w1357 _ w1450 w1508 w1564 w1648 w1724 w1758]
      tunnel: w188 -> [w227 w261 w295 w432 w509 w593 w682 w830 w904 w941 w982 w1026 w1066 w1102 w1129 w1162 w1218 w1260 w1339 w1384 w1437 w1495 w1552 w1642 w1720 w1760]
      tunnel: w187 -> [w226 w260 w286 w403 w494 w562 w651 w801 w872 w942 w983 w1027 w1067 w1103 w1130 w1167 w1220 w1288 w1363 w1388 w1456 w1514 w1570 w1654 w1678 w1764]
      tunnel: w186 -> [w225 w259 w285 w402 w493 w561 w648 w800 w869 w943 w984 w1028 w1068 w1104 w1131 w1166 w1191 w1287 w1362 w1387 w1455 w1513 w1569 w1653 w1677 w1763]
      tunnel: w185 -> [w224 w258 w294 w428 w469 w589 w678 w826 w900 w951 w992 w1025 w1065 w1101 w1128 w1165 w1215 w1251 w1331 w1393 w1430 w1488 w1545 w1641 w1719 w1765]
      tunnel: w184 -> [w223 w257 w293 w430 w507 w591 w680 w828 w902 w950 w991 w1033 w1072 w1107 w1135 w1164 w1200 w1286 w1361 w1396 w1454 w1512 w1568 w1652 w1728 w1766]
      tunnel: w183 -> [w222 w256 w292 w429 w506 w590 w679 w827 w901 w949 w990 w1032 w1071 w1106 w1134 w1163 w1201 w1261 w1340 w1395 w1438 w1496 w1553 w1643 w1721 w1768]
      tunnel: [w226 w260 w284 w427 w504 w587 w677 w825 w898 w942 w983 w1027 w1067 w1103 w1130 w1167 w1220 w1252 w1313 w1386 w1431 w1489 w1546 w1594 w1680 w1764] -> w182
      tunnel: [w225 w259 w283 w426 w503 w586 w676 w824 w897 w943 w984 w1028 w1068 w1104 w1131 w1166 w1190 w1262 w1314 w1385 w1439 w1497 w1554 w1593 w1679 w1762] -> w113
      tunnel: [w224 w258 w294 w428 w465 w589 w678 w826 w900 w944 w985 w1025 w1065 w1101 w1128 w1165 w1215 w1251 w1331 w1393 w1430 w1488 w1545 w1641 w1719 w1765] -> w181
      tunnel: [w223 w257 w293 w430 w507 w591 w680 w828 w902 w950 w991 w1033 w1072 w1107 w1135 w1164 w1200 w1286 w1361 w1396 w1454 w1512 w1568 w1652 w1728 w1766] -> w180
      tunnel: [w222 w256 w292 w429 w506 w590 w679 w827 w901 w949 w990 w1032 w1071 w1106 w1134 w1163 w1201 w1261 w1340 w1395 w1438 w1496 w1553 w1643 w1721 w1768] -> w179
      tunnel: [w227 w261 w295 w432 w509 w593 w682 w830 w904 w941 w982 w1026 w1066 w1102 w1129 w1162 w1218 w1260 w1339 w1384 w1437 w1495 w1552 w1642 w1720 w1760] -> w67
      tunnel: w178 -> [_ _ _ w434 w513 w598 w685 w832 w908 _ _ _ _ _ _ _ _ w1257 w1336 _ w1436 w1494 w1551 w1614 w1696 _]
      tunnel: "Gate" -> [_ _ _ w412 w497 w572 w662 w810 w883 _ _ _ _ _ _ _ _ _ _ _ _ _ _ _ _ _]
      tunnel: "Drain 2" -> [_ _ _ w411 w496 w571 w661 w809 w882 _ _ _ _ _ _ _ _ _ _ _ _ _ _ _ _ _]
      tunnel: "Panel Controls" -> [_ _ _ _ _ w570 w660 w699 w881 _ _ _ _ _ _ _ _ _ _ _ _ _ _ _ _ _]
      tunnel: w174 -> [w221 w255 w291 w396 w487 w555 w646 w794 w867 w948 w989 _ w1064 w1100 w1127 w1161 w1202 w1247 w1327 w1389 w1426 w1484 w1541 w1637 w1715 w1769]
      tunnel: w173 -> [w220 w254 w290 w395 w486 w554 w645 w793 w866 w947 w988 w1031 _ w1091 w1133 w1160 w1203 w1248 w1328 w1390 w1427 w1485 w1542 w1638 w1716 w1770]
      tunnel: w172 -> [w219 w253 w289 w394 w485 w553 w644 w792 w865 w946 w987 w1030 w1070 w1105 _ w1159 w1204 w1249 w1329 w1391 w1428 w1486 w1543 w1639 w1717 w1771]
      tunnel: w171 -> [w218 w252 w288 w393 w484 w552 w647 w791 w868 w945 w986 w1029 w1069 _ w1132 w1158 w1205 w1250 w1330 w1392 w1429 w1487 w1544 w1640 w1718 w1772]
      tunnel: [w221 w255 w291 w396 w487 w555 w646 w794 w867 w948 w989 w1024 w1064 w1100 w1127 w1161 w1202 w1247 w1327 w1389 w1426 w1484 w1541 w1637 w1715 w1769] -> w170
      tunnel: [w220 w254 w290 w395 w486 w554 w645 w793 w866 w947 w988 w1031 w1056 w1091 w1133 w1160 w1203 w1248 w1328 w1390 w1427 w1485 w1542 w1638 w1716 w1770] -> w169
      tunnel: [w219 w253 w289 w394 w485 w553 w644 w792 w865 w946 w987 w1030 w1070 w1105 w1126 w1159 w1204 w1249 w1329 w1391 w1428 w1486 w1543 w1639 w1717 w1771] -> w168
      tunnel: [w218 w252 w288 w393 w484 w552 w647 w791 w868 w945 w986 w1029 w1069 w1092 w1132 w1158 w1205 w1250 w1330 w1392 w1429 w1487 w1544 w1640 w1718 w1772] -> w167
      tunnel: w166 -> [_ _ _ w388 w481 _ w640 w786 _ _ _ _ _ _ _ _ _ _ _ _ _ _ _ _ _ _]
      tunnel: w165 -> [_ _ _ w386 w480 _ _ _ _ _ _ _ _ _ _ _ _ _ _ _ _ _ _ _ _ _]
      tunnel: [w217 w248 w281 w318 w457 w542 w637 w717 w854 w940 w980 w1023 w1055 w1090 w1125 w1157 w1186 w1239 w1296 w1383 w1415 w1477 w1535 w1591 w1673 w1761] -> w79
      tunnel: w164 -> [w217 w248 w281 w383 w457 w542 w637 w782 w854 w940 w980 w1023 w1055 w1090 w1125 w1157 w1186 w1239 w1296 w1383 w1415 w1477 w1535 w1591 w1673 w1761]
      tunnel: w131 -> [_ _ _ w380 w454 w540 w635 w779 w851 _ _ _ _ _ _ _ w1184 w1237 w1309 _ w1412 w1474 w1532 w1588 w1669 _]
      tunnel: w162 -> [_ _ _ w377 w453 w538 w634 w776 w850 _ _ _ _ _ _ _ w1182 w1235 w1308 _ w1411 w1473 w1531 w1587 w1670 _]
      tunnel: w114 -> [_ _ _ w372 _ _ _ w771 _ _ _ _ _ _ _ _ _ _ _ _ _ _ _ _ _ _]
      tunnel: [w216 w247 w280 w326 w456 w541 w636 w725 w853 w939 w979 w1022 w1054 w1089 w1124 w1156 w1185 w1238 w1311 w1382 w1414 w1476 w1534 w1590 w1672 w1767] -> w115
      tunnel: w160 -> [w216 w247 w280 w376 w456 w541 w636 w775 w853 w939 w979 w1022 w1054 w1089 w1124 w1156 w1185 w1238 w1311 w1382 w1414 w1476 w1534 w1590 w1672 w1767]
      tunnel: [w215 w246 w279 w317 w452 w537 w633 w716 w849 w938 w978 w1021 w1053 w1088 w1123 w1155 w1181 w1234 w1295 w1381 w1410 w1472 w1530 w1586 w1668 w1756] -> w78
      tunnel: w136 -> [w215 w246 w279 w370 w452 w537 w633 w769 w849 w938 w978 w1021 w1053 w1088 w1123 w1155 w1181 w1234 w1295 w1381 w1410 w1472 w1530 w1586 w1668 w1756]
      tunnel: [w214 w245 w278 w363 w451 w536 w623 w762 w848 w937 w977 w1020 w1052 w1087 w1122 w1154 w1180 w1233 w1307 w1380 w1409 w1471 w1529 w1585 w1667 w1755] -> w109
      tunnel: w122 -> [w214 w245 w278 w363 w451 w536 w623 w762 w848 w937 w977 w1020 w1052 w1087 w1122 w1154 w1180 w1233 w1307 w1380 w1409 w1471 w1529 w1585 w1667 w1754]
      tunnel: [w213 w244 w277 w362 w450 w535 w622 w761 w847 w936 w976 w1019 w1051 w1086 w1121 w1153 w1179 w1232 w1306 w1379 w1408 w1470 w1528 w1584 w1666 w1740] -> w117
      tunnel: w116 -> [w213 w244 w277 w362 w450 w535 w622 w761 w847 w936 w976 w1019 w1051 w1086 w1121 w1153 w1179 w1232 w1306 w1379 w1408 w1470 w1528 w1584 w1666 w1740]
      tunnel: w114 -> [_ _ _ _ _ _ _ _ _ _ _ _ _ _ _ _ _ _ _ _ _ _ _ _ _ _]
      tunnel: [w212 w243 w276 w361 w449 w534 w621 w760 w846 w935 w975 w1018 w1050 w1085 w1120 w1152 w1178 w1231 w1305 w1378 w1407 w1469 w1527 w1583 w1665 w1739] -> w110
      tunnel: w112 -> [w212 w243 w276 w361 w449 w534 w621 w760 w846 w935 w975 w1018 w1050 w1085 w1120 w1152 w1178 w1231 w1305 w1378 w1407 w1469 w1527 w1583 w1665 w1739]
      tunnel: [w210 w241 w274 w311 w446 w532 w619 w710 w844 w933 w974 w1017 w1048 w1083 w1118 w1150 w1176 w1230 w1304 w1377 w1406 w1468 w1525 w1582 w1664 w1738] -> w72
      tunnel: w100 -> [w210 w241 w274 w357 w446 w532 w619 w756 w844 w933 w974 w1017 w1048 w1083 w1118 w1150 w1176 w1230 w1304 w1377 w1406 w1468 w1525 w1582 w1664 w1738]
      tunnel: [w211 w242 w275 w312 w447 w533 w620 w711 w845 w934 w973 w1016 w1049 w1084 w1119 w1151 w1177 w1229 w1303 w1376 w1405 w1467 w1526 w1581 w1663 w1737] -> w73
      tunnel: w99 -> [w211 w242 w275 w356 w447 w533 w620 w755 w845 w934 w973 w1016 w1049 w1084 w1119 w1151 w1177 w1229 w1303 w1376 w1405 w1467 w1526 w1581 w1663 w1737]
      tunnel: [w203 w234 w267 w316 w443 w530 w617 w715 w842 w926 w971 w1014 w1046 w1081 w1116 w1148 w1169 w1222 w1294 w1375 w1398 w1460 w1518 w1574 w1658 w1730] -> w77
      tunnel: w88 -> [w203 w234 w267 w346 w443 w530 w617 w745 w842 w926 w971 w1014 w1046 w1081 w1116 w1148 w1169 w1222 w1294 w1375 w1398 w1460 w1518 w1574 w1658 w1730]
      tunnel: [w202 w233 w266 w315 w444 w531 w618 w714 w843 w925 w972 w1015 w1047 w1082 w1117 w1149 w1168 w1221 w1293 w1374 w1397 w1459 w1517 w1573 w1657 w1729] -> w76
      tunnel: w87 -> [w202 w233 w266 w345 w444 w531 w618 w744 w843 w925 w972 w1015 w1047 w1082 w1117 w1149 w1168 w1221 w1293 w1374 w1397 w1459 w1517 w1573 w1657 w1729]
      tunnel: [w205 w236 w269 w321 w442 w528 w615 w720 w840 w931 w969 w1012 w1044 w1079 w1114 w1146 w1171 w1224 w1298 w1369 w1400 w1462 w1520 w1576 w1656 w1734] -> w70
      tunnel: w86 -> [w205 w236 w269 w342 w442 w528 w615 w741 w840 w931 w969 w1012 w1044 w1079 w1114 w1146 w1171 w1224 w1298 w1369 w1400 w1462 w1520 w1576 w1656 w1734]
      tunnel: [w204 w235 w268 w319 w445 w529 w616 w718 w841 w932 w970 w1013 w1045 w1080 w1115 w1147 w1170 w1223 w1297 w1368 w1399 w1461 w1519 w1575 w1655 w1733] -> w80
      tunnel: w85 -> [w204 w235 w268 w341 w445 w529 w616 w740 w841 w932 w970 w1013 w1045 w1080 w1115 w1147 w1170 w1223 w1297 w1368 w1399 w1461 w1519 w1575 w1655 w1733]
      tunnel: [w207 w238 w271 w310 w441 w526 w613 w709 w838 w929 w967 w1010 w1042 w1077 w1112 w1144 w1173 w1226 w1300 w1371 w1402 w1464 w1522 w1578 w1660 w1736] -> w71
      tunnel: w84 -> [w207 w238 w271 w338 w441 w526 w613 w737 w838 w929 w967 w1010 w1042 w1077 w1112 w1144 w1173 w1226 w1300 w1371 w1402 w1464 w1522 w1578 w1660 w1736]
      tunnel: [w206 w237 w270 w309 w440 w527 w614 w708 w839 w930 w968 w1011 w1043 w1078 w1113 w1145 w1172 w1225 w1299 w1370 w1401 w1463 w1521 w1577 w1659 w1735] -> w69
      tunnel: w83 -> [w206 w237 w270 w337 w440 w527 w614 w736 w839 w930 w968 w1011 w1043 w1078 w1113 w1145 w1172 w1225 w1299 w1370 w1401 w1463 w1521 w1577 w1659 w1735]
      tunnel: [w209 w240 w273 w314 w439 w524 w611 w713 w836 w927 w965 w1008 w1040 w1075 w1110 w1142 w1175 w1228 w1302 w1373 w1404 w1466 w1524 w1580 w1662 w1732] -> w75
      tunnel: w82 -> [w209 w240 w273 w334 w439 w524 w611 w733 w836 w927 w965 w1008 w1040 w1075 w1110 w1142 w1175 w1228 w1302 w1373 w1404 w1466 w1524 w1580 w1662 w1732]
      tunnel: [w208 w239 w272 w313 w438 w525 w612 w712 w837 w928 w966 w1009 w1041 w1076 w1111 w1143 w1174 w1227 w1301 w1372 w1403 w1465 w1523 w1579 w1661 w1731] -> w74
      tunnel: w81 -> [w208 w239 w272 w333 w438 w525 w612 w732 w837 w928 w966 w1009 w1041 w1076 w1111 w1143 w1174 w1227 w1301 w1372 w1403 w1465 w1523 w1579 w1661 w1731]
      frame "wait" {
        n32 = Index Array(array=w232, index=0 ("Index")) -> (element=w230:string)
        n33 = Decimal String To Number(string=w230, default (0L)=u32 0) -> (number=w229:u32)  [unwired: 1 in, 1 out]
        n34 = Wait (ms)(milliseconds to wait=w229) -> ()  [unwired: 1 out]
      }
      frame "wait-min" {
        n35 = Index Array(array=w265, index=0 ("Index")) -> (element=w263:string)
        n36 = Decimal String To Number(string=w263, default (0L)=u32 0) -> (number=w251:u32)  [unwired: 1 in, 1 out]
        n37 = Multiply(x=w251, y=u32 60000) -> (x*y=w250:u32)
        n38 = Wait (ms)(milliseconds to wait=w250) -> ()  [unwired: 1 out]
      }
      frame "standby" {
        n39 = Index Array(array=w297, index=0 ("Index")) -> (element=w287:string)
        n40 = case shown="\"off\", Default" w287 {
          tunnel: [":PAGE:SCON:STAN 0" ":PAGE:SCON:STAN 1"] -> w282
          frame "off", Default {
          }
          frame "on" {
          }
        }
        n41 = VISA Write(VISA resource name=w286, write buffer=w282, error in (no error)=w285) -> (VISA resource name out=w284:refnum<visa-resource-name>, error out=w283:errorcluster)  [unwired: 1 out]
      }
      frame "transfer" {
        # "Adjusts graph colors."
        # "Adjusts graph colors."
        # "Is off"
        # "Is on"
        # "Ion will be the middle element of the array. The calculation of the index is done only once, since Is, Id, and Ig have the same dimensions."
        # "Ig off"
        # "Ig on"
        # "Is min"
        # "Is max"
        # "Ig min"
        # "Ig max"
        # "abs(Ig)"
        # "abs(Is)"
        # "Id min"
        # "Id max"
        # "Y1: Is\nY2: Id\nY3: Ig"
        # "abs(Id)"
        # "Adjusts graph colors."
        # "Adjusts graph colors."
        # "Id off"
        # "Id on"
        # "Adjusts graph colors."
        # "Time array"
        n42 = Delete From Array(array=w425, index=0 ("Index")) -> (deleted portion=w423:string, array with subset deleted=w422:string[])  [unwired: 1 in]
        n43 = Bundle By Name(cluster=w386, "Emergency Stop"=w434) -> (w387:T3)
        n44 = Number To Decimal String(number=w380) -> (decimal integer string=w379:string)  [unwired: 1 in]
        n45 = case shown="\"d\", Default" w423 {
          tunnel: [w436 w437] -> w421
          frame "s" {
            w436 = u16 0 items=["Single", "Double"] ("sweep mode")
          }
          frame "d", Default {
            w437 = u16 1 items=["Single", "Double"] ("sweep mode")
          }
        }
        n46 = Fract/Exp String To Number(string=w422) -> (number=w407:dbl[])  [unwired: 3 in, 1 out]
        n47 = Concatenate Strings(w432, "-transfer-" ("Prefix"), w379, w377, ".txt" ("Suffix (transfer)")) -> (w433:string)
        n48 = VISA Write(VISA resource name=w403, write buffer=":PAGE:CHAN:MODE SWE;" ("write buffer (\"\")"), error in (no error)=w402) -> (VISA resource name out=w400:refnum<visa-resource-name>, error out=w401:errorcluster)  [unwired: 1 out]
        n49 = String To Path(string=w433) -> (path=w431:path)
        n50 = Index Array(array=w407, index #1=0 ("Index")) -> (element #1=w420:dbl, element #2=w419:dbl, element #3=w418:dbl)  [unwired: 2 in]
        n51 = Delete From Array(array=w407, length=3 ("Length"), index=0 ("Index")) -> (array with subset deleted=w405:dbl[])  [unwired: 1 out]
        n52 = Build Array (concatenate)(w376, w372) -> (w326:i32[])
        n53 = Bundle By Name(cluster=w412, "Gate Start"=w420, "Gate Stop"=w419, "Gate Step (linear only)"=w418, "Gate Compliance"=w429, "Range mode"=w396, "Range"=w395) -> (w397:T6)
        n54 = control-ref of="Imax vs time"() -> (w355:refnum<vi>)
        n55 = control-ref of="Imin vs time"() -> (w354:refnum<vi>)
        n56 = control-ref of="Ion vs time"() -> (w323:refnum<vi>)
        n57 = control-ref of="Ioff vs time"() -> (w322:refnum<vi>)
        n58 = control-ref of="I vs Vg"() -> (w381:refnum<vi>)
        n59 = Index Array(array=w405, index #1=0 ("Index")) -> (element #1=w415:dbl, element #2=w414:dbl, element #3=w413:dbl)  [unwired: 2 in]
        n60 = call <vilib>:"compatOverwrite.vi"("overwrite (F)"=TRUE) -> ("overwrite?"=w385:T8)
        n61 = Bundle By Name(cluster=w411, "Drain Start"=w415, "Drain Stop"=w414, "Drain Step"=w413, "Drain Compliance"=w430, "Range mode"=w394, "Range"=w393) -> (w398:T7)
        n62 = call "4155C Transfer.vi"("VISA resource name in"=w400, "Gate"=w397, "Drain"=w398, "Timings"=w428, "error in (no error)"=w401, "SMU4"=w388, "sweep mode"=w421, "Panel Controls"=w387) -> ("VG"=w384:dbl[], "Outparams"=w392:T9, "VISA Resource Name out"=w427:refnum<visa-resource-name>, "IS"=w351:dbl[], "ID"=w353:dbl[], "IG"=w350:dbl[], "error out"=w373:errorcluster, "SMU4"=w389:dbl[])  [unwired: 12 in]
        n63 = Unbundle By Name(w392) -> ("V2 Step"=w391:dbl, "V2 Start"=w390:dbl, "Number of points"=w320:i32)
        n64 = Absolute Value(x=w351) -> (abs(x)=w336:dbl[])
        n65 = Absolute Value(x=w353) -> (abs(x)=w352:dbl[])
        n66 = Absolute Value(x=w350) -> (abs(x)=w339:dbl[])
        n67 = Array Size(array=w352) -> (size(s)=w360:i32)
        n68 = Divide(x=w360, y=2) -> (x/y=w303:dbl)
        n69 = Subtract(x=w303, y=1) -> (x-y=w302:dbl)
        n70 = Array Max & Min(array=w336) -> (max value=w343:dbl, min value=w344:dbl)  [unwired: 2 out]
        n71 = Array Max & Min(array=w352) -> (max value=w382:dbl, min value=w349:dbl)  [unwired: 2 out]
        n72 = Array Max & Min(array=w339) -> (max value=w348:dbl, min value=w347:dbl)  [unwired: 2 out]
        n73 = call "4155C Split array.vi"("Number of VAR2 steps"=w320, "Y2 data in"=w353, "X data in"=w384, "Y1 data in"=w351, "Y3 data in"=w350, "error in (no error)"=w373) -> ("Array of clusters"=w375:cluster{"Y data in":dbl[], "X data in":dbl[]}[], "error out"=w308:errorcluster)  [unwired: 1 in]
        n74 = Index Array(array=w336, index=w302) -> (element=w327:dbl)
        n75 = Index Array(array=w336, index=0) -> (element=w328:dbl)
        n76 = Index Array(array=w352, index=w302) -> (element=w329:dbl)
        n77 = Index Array(array=w352, index=0) -> (element=w330:dbl)
        n78 = Index Array(array=w339, index=w302) -> (element=w332:dbl)
        n79 = Index Array(array=w339, index=0) -> (element=w331:dbl)
        n80 = local write "Ig max"(w348) -> ()
        n81 = local write "Ig min"(w347) -> ()
        n82 = local write "Is max"(w343) -> ()
        n83 = local write "Is min"(w344) -> ()
        n84 = local write "Id max"(w382) -> ()
        n85 = local write "Id min"(w349) -> ()
        n86 = local write "I vs Vg"(w375) -> ()
        n87 = Build Array (concatenate)(w342, w343) -> (w321:dbl[])
        n88 = Build Array (concatenate)(w341, w344) -> (w319:dbl[])
        n89 = local write "Is off"(w328) -> ()
        n90 = local write "Is on"(w327) -> ()
        n91 = Build Array (concatenate)(w383, w382) -> (w318:dbl[])
        n92 = Build Array (concatenate)(w370, w349) -> (w317:dbl[])
        n93 = Build Array (concatenate)(w346, w348) -> (w316:dbl[])
        n94 = Build Array (concatenate)(w345, w347) -> (w315:dbl[])
        n95 = Build Array (concatenate)(w334, w327) -> (w314:dbl[])
        n96 = Build Array (concatenate)(w333, w328) -> (w313:dbl[])
        n97 = Build Array (concatenate)(w356, w329) -> (w312:dbl[])
        n98 = Build Array (concatenate)(w357, w330) -> (w311:dbl[])
        n99 = Build Array (concatenate)(w338, w332) -> (w310:dbl[])
        n100 = Build Array (concatenate)(w337, w331) -> (w309:dbl[])
        n101 = local write "Ig off"(w331) -> ()
        n102 = local write "Ig on"(w332) -> ()
        n103 = local write "Id off"(w330) -> ()
        n104 = local write "Id on"(w329) -> ()
        n105 = call "4155C Split array.vi"("Number of VAR2 steps"=w320, "Y2 data in"=w312, "X data in"=w326, "Y1 data in"=w314, "Y3 data in"=w310, "error in (no error)"=w308) -> ("Array of clusters"=w324:cluster{"Y data in":dbl[], "X data in":dbl[]}[], "error out"=w307:errorcluster)  [unwired: 1 in]
        n106 = call "4155C Split array.vi"("Number of VAR2 steps"=w320, "Y2 data in"=w311, "X data in"=w326, "Y1 data in"=w313, "Y3 data in"=w309, "error in (no error)"=w307) -> ("Array of clusters"=w325:cluster{"Y data in":dbl[], "X data in":dbl[]}[], "error out"=w306:errorcluster)  [unwired: 1 in]
        n107 = call "4155C Split array.vi"("Number of VAR2 steps"=w320, "Y2 data in"=w318, "X data in"=w326, "Y1 data in"=w321, "Y3 data in"=w316, "error in (no error)"=w306) -> ("Array of clusters"=w374:cluster{"Y data in":dbl[], "X data in":dbl[]}[], "error out"=w305:errorcluster)  [unwired: 1 in]
        n108 = call "4155C Split array.vi"("Number of VAR2 steps"=w320, "Y2 data in"=w317, "X data in"=w326, "Y1 data in"=w319, "Y3 data in"=w315, "error in (no error)"=w305) -> ("Array of clusters"=w371:cluster{"Y data in":dbl[], "X data in":dbl[]}[], "error out"=w304:errorcluster)  [unwired: 1 in]
        n109 = Open/Create/Replace File(file path (use dialog)=w431, error in=w304, operation (0:open)=w385) -> (refnum out=w368:refnum<file>, error out=w366:errorcluster)  [unwired: 3 in, 1 out]
        n110 = call "4155C Make Big 2d array.vi"("1D Var1"=w384, "1d IS"=w351, "1d ID"=w353, "1d IG"=w350, "1d SMU4"=w389, "SMU4"=w388, "VAR2 START"=w390, "Number of VAR2 steps"=w320, "VAR2 STEP"=w391, "VAR1 Name"="Vg", "Decimal places in header"=i8 1, "VAR2 Name"="Vd") -> ("Header array"=w369:string[], "Data array"=w367:dbl[][])  [unwired: 14 in]
        n111 = local write "Imax vs time"(w374) -> ()
        n112 = local write "Imin vs time"(w371) -> ()
        n113 = local write "Ion vs time"(w324) -> ()
        n114 = local write "Ioff vs time"(w325) -> ()
        n115 = call "4155C Config Chart Colours.vi"("Numeric"=w320, "XY Graph 2"=w355) -> ()  [unwired: 6 in]
        n116 = call "4155C Config Chart Colours.vi"("Numeric"=w320, "XY Graph 2"=w354) -> ()  [unwired: 6 in]
        n117 = call "4155C Config Chart Colours.vi"("Numeric"=w320, "XY Graph 2"=w323) -> ()  [unwired: 6 in]
        n118 = call "4155C Config Chart Colours.vi"("Numeric"=w320, "XY Graph 2"=w322) -> ()  [unwired: 6 in]
        n119 = call "4155C Config Chart Colours.vi"("Numeric"=w320, "XY Graph 2"=w381) -> ()  [unwired: 6 in]
        n120 = call "4155C Write array to file.vi"("Byte Stream File Refnum"=w368, "Header"=w369, "Data Array"=w367, "error in (no error)"=w366) -> ("dup refnum"=w365:refnum<file>, "error out"=w364:errorcluster)  [unwired: 1 in]
        n121 = Close File(refnum=w365, error in=w364) -> (error out=w426:errorcluster)  [unwired: 1 out]
      }
      frame "pulsedstressV" {
        w463 = 0
        n122 = Number To Decimal String(number=w454) -> (decimal integer string=w510:string)  [unwired: 1 in]
        n123 = Delete From Array(array=w448, index=0 ("Index")) -> (deleted portion=w501:string, array with subset deleted=w500:string[])  [unwired: 1 in]
        n124 = Bundle By Name(cluster=w480, "Emergency Stop"=w513) -> (w482:T3)
        n125 = VISA Write(VISA resource name=w494, write buffer=":PAGE:CHAN:MODE SWE;" ("write buffer (\"\")"), error in (no error)=w493) -> (VISA resource name out=w491:refnum<visa-resource-name>, error out=w492:errorcluster)  [unwired: 1 out]
        n126 = Concatenate Strings(w509, "-pulsedstressV-" ("Substring"), w510, w453, ".txt" ("Substring")) -> (w512:string)
        n127 = case shown="\"d\", Default" w501 {
          tunnel: [w522 w523] -> w499
          frame "s" {
            w522 = u16 0 items=["Single", "Double"] ("sweep mode")
          }
          frame "d", Default {
            w523 = u16 1 items=["Single", "Double"] ("sweep mode")
          }
        }
        n128 = Fract/Exp String To Number(string=w500) -> (number=w495:dbl[])  [unwired: 3 in, 1 out]
        n129 = String To Path(string=w512) -> (path=w508:path)
        n130 = Index Array(array=w495, index #1=0 ("Index")) -> (element #1=w472:dbl, element #2=w471:dbl, element #3=w468:dbl, element #4=w467:dbl, element #5=w466:dbl, element #6=w470:dbl)  [unwired: 5 in]
        n131 = Bundle By Name(cluster=w469, "Pulse period"=w467, "Base voltage"=w468, "Pulse width"=w466) -> (w465:T5)
        n132 = Unbundle By Name(w465) -> ("Pulse period"=w473:dbl)
        n133 = Bundle By Name(cluster=w497, "Gate Start"=w471, "Gate Stop"=w472, "Gate Step (linear only)"=0, "Gate Compliance"=w506, "Range mode"=w487, "Range"=w486) -> (w488:T6)
        n134 = call <vilib>:"compatOverwrite.vi"("overwrite (F)"=TRUE) -> ("overwrite?"=w458:T8)
        n135 = Bundle By Name(cluster=w496, "Drain Start"=w470, "Drain Stop"=w463, "Drain Step"=w463, "Drain Compliance"=w507, "Range mode"=w485, "Range"=w484) -> (w489:T7)
        n136 = call "4155C PulsedStressV.vi"("VISA resource name in"=w491, "sweep mode"=w499, "Panel Controls"=w482, "Gate"=w488, "Drain"=w489, "Timings"=w465, "error in (no error)"=w492, "SMU4"=w481) -> ("VISA Resource Name out"=w504:refnum<visa-resource-name>, "ID"=w461:dbl[], "IG"=w459:dbl[], "Outparams"=w483:T9, "error out"=w505:errorcluster)  [unwired: 3 in]
        n137 = Unbundle By Name(w483) -> ("Number of points"=w460:i32)  [unwired: 2 out]
        n138 = for {
          N: w460 -> [_]
          tunnel: [w519] -> w462 mode=indexing
          tunnel: w473 -> [w521]
          i -> [w520]
          n139 = Multiply(x=w521, y=w520) -> (x*y=w519:dbl)
        }
        n140 = Insert Into Array(array=dbl[][] [] ("Input Array"), new element=w462) -> (w474:dbl[][])  [unwired: 2 in]
        n141 = Insert Into Array(array=w474, new element=w461) -> (w479:dbl[][])  [unwired: 2 in]
        n142 = Insert Into Array(array=w479, new element=w459) -> (w478:dbl[][])  [unwired: 2 in]
        n143 = Transpose 2D Array(2D array=w478) -> (transposed array=w477:dbl[][])
        n144 = Open/Create/Replace File(file path (use dialog)=w508, error in=w505, operation (0:open)=w458) -> (refnum out=w516:refnum<file>, error out=w517:errorcluster)  [unwired: 3 in, 1 out]
        n145 = call "4155C Write array to file.vi"("Byte Stream File Refnum"=w516, "Header"=string[] ["Time /s", "Id /A", "Ig /A"], "Data Array"=w477, "error in (no error)"=w517) -> ("dup refnum"=w514:refnum<file>, "error out"=w515:errorcluster)  [unwired: 1 in]
        n146 = Close File(refnum=w514, error in=w515) -> (error out=w503:errorcluster)  [unwired: 1 out]
      }
      frame "transfer-fpp" {
        n147 = Number To Decimal String(number=w540) -> (decimal integer string=w594:string)  [unwired: 1 in]
        n148 = Bundle By Name(cluster=w570, "Emergency Stop"=w598) -> (w606:T2)
        n149 = Delete From Array(array=w585, index=0 ("Index")) -> (deleted portion=w583:string, array with subset deleted=w582:string[])  [unwired: 1 in]
        n150 = Concatenate Strings(w593, "-transferfpp-" ("Substring"), w594, w538, ".txt" ("Substring")) -> (w596:string)
        n151 = VISA Write(VISA resource name=w562, write buffer=":PAGE:CHAN:MODE SWE;" ("write buffer (\"\")"), error in (no error)=w561) -> (VISA resource name out=w559:refnum<visa-resource-name>, error out=w560:errorcluster)  [unwired: 1 out]
        n152 = case shown="\"d\", Default" w583 {
          tunnel: [w607 w608] -> w581
          frame "s" {
            w607 = u16 0 items=["Single", "Double"] ("sweep mode")
          }
          frame "d", Default {
            w608 = u16 1 items=["Single", "Double"] ("sweep mode")
          }
        }
        n153 = Fract/Exp String To Number(string=w582) -> (number=w566:dbl[])  [unwired: 3 in, 1 out]
        n154 = String To Path(string=w596) -> (path=w592:path)
        n155 = Index Array(array=w566, index #1=0 ("Index")) -> (element #1=w580:dbl, element #2=w579:dbl, element #3=w578:dbl)  [unwired: 2 in]
        n156 = Delete From Array(array=w566, length=3 ("Length"), index=0 ("Index")) -> (array with subset deleted=w564:dbl[])  [unwired: 1 out]
        n157 = Bundle By Name(cluster=w572, "Gate Start"=w580, "Gate Stop"=w579, "Gate Step (linear only)"=w578, "Gate Compliance"=w590, "Range mode"=w555, "Range"=w554) -> (w556:T6)
        n158 = Index Array(array=w564, index #1=0 ("Index")) -> (element #1=w575:dbl, element #2=w574:dbl, element #3=w573:dbl)  [unwired: 2 in]
        n159 = call <vilib>:"compatOverwrite.vi"("overwrite (F)"=TRUE) -> ("overwrite?"=w543:T8)
        n160 = Bundle By Name(cluster=w571, "Drain Start"=w575, "Drain Stop"=w574, "Drain Step"=w573, "Drain Compliance"=w591, "Range mode"=w553, "Range"=w552) -> (w557:T7)
        n161 = call "4155C Transfer-FPP.vi"("VISA resource name in"=w559, "Gate"=w556, "Drain"=w557, "Timings"=w589, "error in (no error)"=w560, "sweep mode"=w581, "Panel Controls"=w606) -> ("VG"=w597:dbl[], "Outparams"=w551:T9, "VISA Resource Name out"=w587:refnum<visa-resource-name>, "Vprobe2"=w547:dbl[], "ID"=w546:dbl[], "IG"=w545:dbl[], "Vprobe1"=w544:dbl[], "error out"=w588:errorcluster)  [unwired: 13 in]
        n162 = Unbundle By Name(w551) -> ("V2 Step"=w550:dbl, "V2 Start"=w549:dbl, "Number of points"=w548:i32)
        n163 = Open/Create/Replace File(file path (use dialog)=w592, error in=w588, operation (0:open)=w543) -> (refnum out=w603:refnum<file>, error out=w604:errorcluster)  [unwired: 3 in, 1 out]
        n164 = call "4155C Make Big 2d array FPP.vi"("1D Var1"=w597, "1d ID"=w546, "1d Vp2"=w547, "1d IG"=w545, "1d Vp1"=w544, "VAR2 START"=w549, "Number of VAR2 steps"=w548, "VAR2 STEP"=w550, "VAR1 Name"="Vg", "Decimal places in header"=i8 1, "VAR2 Name"="Vd") -> ("Header array"=w599:string[], "Data array"=w600:dbl[][])  [unwired: 15 in]
        n165 = call "4155C Write array to file.vi"("Byte Stream File Refnum"=w603, "Header"=w599, "Data Array"=w600, "error in (no error)"=w604) -> ("dup refnum"=w601:refnum<file>, "error out"=w602:errorcluster)  [unwired: 1 in]
        n166 = Close File(refnum=w601, error in=w602) -> (error out=w586:errorcluster)  [unwired: 1 out]
      }
      frame "output" {
        n167 = Number To Decimal String(number=w635) -> (decimal integer string=w683:string)  [unwired: 1 in]
        n168 = Bundle By Name(cluster=w660, "Emergency Stop"=w685) -> (w695:T2)
        n169 = Delete From Array(array=w675, index=0 ("Index")) -> (deleted portion=w673:string, array with subset deleted=w672:string[])  [unwired: 1 in]
        n170 = Concatenate Strings(w682, "-output-" ("Substring"), w683, w634, ".txt" ("Suffix (output)")) -> (w684:string)
        n171 = VISA Write(VISA resource name=w651, write buffer=":PAGE:CHAN:MODE SWE;" ("write buffer (\"\")"), error in (no error)=w648) -> (VISA resource name out=w650:refnum<visa-resource-name>, error out=w649:errorcluster)  [unwired: 1 out]
        n172 = case shown="\"d\", Default" w673 {
          tunnel: [w696 w697] -> w671
          frame "s" {
            w696 = u16 0 items=["Single", "Double"] ("sweep mode")
          }
          frame "d", Default {
            w697 = u16 1 items=["Single", "Double"] ("sweep mode")
          }
        }
        n173 = Fract/Exp String To Number(string=w672) -> (number=w654:dbl[])  [unwired: 3 in, 1 out]
        n174 = String To Path(string=w684) -> (path=w681:path)
        n175 = Index Array(array=w654, index #1=0 ("Index")) -> (element #1=w670:dbl, element #2=w669:dbl, element #3=w668:dbl)  [unwired: 2 in]
        n176 = Delete From Array(array=w654, length=3 ("Length"), index=0 ("Index")) -> (array with subset deleted=w653:dbl[])  [unwired: 1 out]
        n177 = control-ref of="I vs Vd"() -> (w625:refnum<vi>)
        n178 = Bundle By Name(cluster=w662, "Gate Start"=w670, "Gate Stop"=w669, "Gate Step (linear only)"=w668, "Gate Compliance"=w679, "Range mode"=w646, "Range"=w645) -> (w694:T6)
        n179 = Index Array(array=w653, index #1=0 ("Index")) -> (element #1=w665:dbl, element #2=w664:dbl, element #3=w663:dbl)  [unwired: 2 in]
        n180 = call <vilib>:"compatOverwrite.vi"("overwrite (F)"=TRUE) -> ("overwrite?"=w638:T8)
        n181 = Bundle By Name(cluster=w661, "Drain Start"=w665, "Drain Stop"=w664, "Drain Step"=w663, "Drain Compliance"=w680, "Range mode"=w644, "Range"=w647) -> (w693:T7)
        n182 = call "4155C Output.vi"("VISA resource name in"=w650, "Gate"=w694, "Drain"=w693, "Timings"=w678, "error in (no error)"=w649, "SMU4"=w640, "sweep mode"=w671, "Panel controls"=w695) -> ("VD"=w632:dbl[], "Outparams"=w642:T9, "VISA Resource Name out"=w677:refnum<visa-resource-name>, "IS"=w631:dbl[], "ID"=w630:dbl[], "IG"=w629:dbl[], "error out"=w627:errorcluster, "SMU4"=w639:dbl[])  [unwired: 12 in]
        n183 = Unbundle By Name(w642) -> ("V2 Step"=w643:dbl, "V2 Start"=w641:dbl, "Number of points"=w624:i32)
        n184 = call "4155C Split array.vi"("Number of VAR2 steps"=w624, "Y2 data in"=w630, "X data in"=w632, "Y1 data in"=w631, "Y3 data in"=w629, "error in (no error)"=w627) -> ("Array of clusters"=w628:cluster{"Y data in":dbl[], "X data in":dbl[]}[], "error out"=w626:errorcluster)  [unwired: 1 in]
        n185 = local write "I vs Vd"(w628) -> ()
        n186 = call "4155C Config Chart Colours.vi"("Numeric"=w624, "XY Graph 2"=w625) -> ()  [unwired: 6 in]
        n187 = Open/Create/Replace File(file path (use dialog)=w681, error in=w626, operation (0:open)=w638) -> (refnum out=w690:refnum<file>, error out=w691:errorcluster)  [unwired: 3 in, 1 out]
        n188 = call "4155C Make Big 2d array.vi"("1D Var1"=w632, "1d IS"=w631, "1d ID"=w630, "1d IG"=w629, "1d SMU4"=w639, "SMU4"=w640, "VAR2 START"=w641, "Number of VAR2 steps"=w624, "VAR2 STEP"=w643, "VAR1 Name"="Vd", "Decimal places in header"=i8 1, "VAR2 Name"="Vg") -> ("Header array"=w686:string[], "Data array"=w687:dbl[][])  [unwired: 14 in]
        n189 = call "4155C Write array to file.vi"("Byte Stream File Refnum"=w690, "Header"=w686, "Data Array"=w687, "error in (no error)"=w691) -> ("dup refnum"=w688:refnum<file>, "error out"=w689:errorcluster)  [unwired: 1 in]
        n190 = Close File(refnum=w688, error in=w689) -> (error out=w676:errorcluster)  [unwired: 1 out]
      }
      frame "output2" {
        # "Adjusts graph colors."
        # "Adjusts graph colors."
        # "Is off"
        # "Is on"
        # "Ion will be the middle element of the array. The calculation of the index is done only once, since Is, Id, and Ig have the same dimensions."
        # "Ig off"
        # "Ig on"
        # "Is min"
        # "Is max"
        # "Ig min"
        # "Ig max"
        # "abs(Ig)"
        # "abs(Is)"
        # "Id min"
        # "Id max"
        # "Y1: Is\nY2: Id\nY3: Ig"
        # "abs(Id)"
        # "Adjusts graph colors."
        # "Adjusts graph colors."
        # "Id off"
        # "Id on"
        # "Adjusts graph colors."
        # "Time array"
        n191 = Delete From Array(array=w823, index=0 ("Index")) -> (deleted portion=w821:string, array with subset deleted=w820:string[])  [unwired: 1 in]
        n192 = Bundle By Name(cluster=w699, "Emergency Stop"=w832) -> (w785:T2)
        n193 = Number To Decimal String(number=w779) -> (decimal integer string=w778:string)  [unwired: 1 in]
        n194 = case shown="\"d\", Default" w821 {
          tunnel: [w834 w835] -> w819
          frame "s" {
            w834 = u16 0 items=["Single", "Double"] ("sweep mode")
          }
          frame "d", Default {
            w835 = u16 1 items=["Single", "Double"] ("sweep mode")
          }
        }
        n195 = Fract/Exp String To Number(string=w820) -> (number=w805:dbl[])  [unwired: 3 in, 1 out]
        n196 = Concatenate Strings(w830, "-output-" ("Substring"), w778, w776, ".txt" ("Suffix (transfer)")) -> (w831:string)
        n197 = VISA Write(VISA resource name=w801, write buffer=":PAGE:CHAN:MODE SWE;" ("write buffer (\"\")"), error in (no error)=w800) -> (VISA resource name out=w798:refnum<visa-resource-name>, error out=w799:errorcluster)  [unwired: 1 out]
        n198 = String To Path(string=w831) -> (path=w829:path)
        n199 = Index Array(array=w805, index #1=0 ("Index")) -> (element #1=w818:dbl, element #2=w817:dbl, element #3=w816:dbl)  [unwired: 2 in]
        n200 = Delete From Array(array=w805, length=3 ("Length"), index=0 ("Index")) -> (array with subset deleted=w803:dbl[])  [unwired: 1 out]
        n201 = Build Array (concatenate)(w775, w771) -> (w725:i32[])
        n202 = Bundle By Name(cluster=w810, "Gate Start"=w818, "Gate Stop"=w817, "Gate Step (linear only)"=w816, "Gate Compliance"=w827, "Range mode"=w794, "Range"=w793) -> (w795:T6)
        n203 = control-ref of="Imax vs time"() -> (w754:refnum<vi>)
        n204 = control-ref of="Imin vs time"() -> (w753:refnum<vi>)
        n205 = control-ref of="Ion vs time"() -> (w722:refnum<vi>)
        n206 = control-ref of="Ioff vs time"() -> (w721:refnum<vi>)
        n207 = control-ref of="I vs Vg"() -> (w780:refnum<vi>)
        n208 = Index Array(array=w803, index #1=0 ("Index")) -> (element #1=w813:dbl, element #2=w812:dbl, element #3=w811:dbl)  [unwired: 2 in]
        n209 = call <vilib>:"compatOverwrite.vi"("overwrite (F)"=TRUE) -> ("overwrite?"=w784:T8)
        n210 = Bundle By Name(cluster=w809, "Drain Start"=w813, "Drain Stop"=w812, "Drain Step"=w811, "Drain Compliance"=w828, "Range mode"=w792, "Range"=w791) -> (w796:T7)
        n211 = call "4155C Output.vi"("VISA resource name in"=w798, "Gate"=w795, "Drain"=w796, "Timings"=w826, "error in (no error)"=w799, "SMU4"=w786, "sweep mode"=w819, "Panel controls"=w785) -> ("VD"=w783:dbl[], "Outparams"=w790:T9, "VISA Resource Name out"=w825:refnum<visa-resource-name>, "IS"=w750:dbl[], "ID"=w752:dbl[], "IG"=w749:dbl[], "error out"=w772:errorcluster, "SMU4"=w787:dbl[])  [unwired: 12 in]
        n212 = Unbundle By Name(w790) -> ("V2 Step"=w789:dbl, "V2 Start"=w788:dbl, "Number of points"=w719:i32)
        n213 = Absolute Value(x=w750) -> (abs(x)=w735:dbl[])
        n214 = Absolute Value(x=w752) -> (abs(x)=w751:dbl[])
        n215 = Absolute Value(x=w749) -> (abs(x)=w738:dbl[])
        n216 = Array Size(array=w751) -> (size(s)=w759:i32)
        n217 = Divide(x=w759, y=2) -> (x/y=w702:dbl)
        n218 = Subtract(x=w702, y=1) -> (x-y=w701:dbl)
        n219 = Array Max & Min(array=w735) -> (max value=w742:dbl, min value=w743:dbl)  [unwired: 2 out]
        n220 = Array Max & Min(array=w751) -> (max value=w781:dbl, min value=w748:dbl)  [unwired: 2 out]
        n221 = Array Max & Min(array=w738) -> (max value=w747:dbl, min value=w746:dbl)  [unwired: 2 out]
        n222 = call "4155C Split array.vi"("Number of VAR2 steps"=w719, "Y2 data in"=w752, "X data in"=w783, "Y1 data in"=w750, "Y3 data in"=w749, "error in (no error)"=w772) -> ("Array of clusters"=w774:cluster{"Y data in":dbl[], "X data in":dbl[]}[], "error out"=w707:errorcluster)  [unwired: 1 in]
        n223 = Index Array(array=w735, index=w701) -> (element=w726:dbl)
        n224 = Index Array(array=w735, index=0) -> (element=w727:dbl)
        n225 = Index Array(array=w751, index=w701) -> (element=w728:dbl)
        n226 = Index Array(array=w751, index=0) -> (element=w729:dbl)
        n227 = Index Array(array=w738, index=w701) -> (element=w731:dbl)
        n228 = Index Array(array=w738, index=0) -> (element=w730:dbl)
        n229 = local write "Ig max"(w747) -> ()
        n230 = local write "Ig min"(w746) -> ()
        n231 = local write "Is max"(w742) -> ()
        n232 = local write "Is min"(w743) -> ()
        n233 = local write "Id max"(w781) -> ()
        n234 = local write "Id min"(w748) -> ()
        n235 = local write "I vs Vd"(w774) -> ()
        n236 = Build Array (concatenate)(w741, w742) -> (w720:dbl[])
        n237 = Build Array (concatenate)(w740, w743) -> (w718:dbl[])
        n238 = local write "Is off"(w727) -> ()
        n239 = local write "Is on"(w726) -> ()
        n240 = Build Array (concatenate)(w782, w781) -> (w717:dbl[])
        n241 = Build Array (concatenate)(w769, w748) -> (w716:dbl[])
        n242 = Build Array (concatenate)(w745, w747) -> (w715:dbl[])
        n243 = Build Array (concatenate)(w744, w746) -> (w714:dbl[])
        n244 = Build Array (concatenate)(w733, w726) -> (w713:dbl[])
        n245 = Build Array (concatenate)(w732, w727) -> (w712:dbl[])
        n246 = Build Array (concatenate)(w755, w728) -> (w711:dbl[])
        n247 = Build Array (concatenate)(w756, w729) -> (w710:dbl[])
        n248 = Build Array (concatenate)(w737, w731) -> (w709:dbl[])
        n249 = Build Array (concatenate)(w736, w730) -> (w708:dbl[])
        n250 = local write "Ig off"(w730) -> ()
        n251 = local write "Ig on"(w731) -> ()
        n252 = local write "Id off"(w729) -> ()
        n253 = local write "Id on"(w728) -> ()
        n254 = call "4155C Split array.vi"("Number of VAR2 steps"=w719, "Y2 data in"=w711, "X data in"=w725, "Y1 data in"=w713, "Y3 data in"=w709, "error in (no error)"=w707) -> ("Array of clusters"=w723:cluster{"Y data in":dbl[], "X data in":dbl[]}[], "error out"=w706:errorcluster)  [unwired: 1 in]
        n255 = call "4155C Split array.vi"("Number of VAR2 steps"=w719, "Y2 data in"=w710, "X data in"=w725, "Y1 data in"=w712, "Y3 data in"=w708, "error in (no error)"=w706) -> ("Array of clusters"=w724:cluster{"Y data in":dbl[], "X data in":dbl[]}[], "error out"=w705:errorcluster)  [unwired: 1 in]
        n256 = call "4155C Split array.vi"("Number of VAR2 steps"=w719, "Y2 data in"=w717, "X data in"=w725, "Y1 data in"=w720, "Y3 data in"=w715, "error in (no error)"=w705) -> ("Array of clusters"=w773:cluster{"Y data in":dbl[], "X data in":dbl[]}[], "error out"=w704:errorcluster)  [unwired: 1 in]
        n257 = call "4155C Split array.vi"("Number of VAR2 steps"=w719, "Y2 data in"=w716, "X data in"=w725, "Y1 data in"=w718, "Y3 data in"=w714, "error in (no error)"=w704) -> ("Array of clusters"=w770:cluster{"Y data in":dbl[], "X data in":dbl[]}[], "error out"=w703:errorcluster)  [unwired: 1 in]
        n258 = Open/Create/Replace File(file path (use dialog)=w829, error in=w703, operation (0:open)=w784) -> (refnum out=w767:refnum<file>, error out=w765:errorcluster)  [unwired: 3 in, 1 out]
        n259 = call "4155C Make Big 2d array.vi"("1D Var1"=w783, "1d IS"=w750, "1d ID"=w752, "1d IG"=w749, "1d SMU4"=w787, "SMU4"=w786, "VAR2 START"=w788, "Number of VAR2 steps"=w719, "VAR2 STEP"=w789, "VAR1 Name"="Vd", "Decimal places in header"=i8 1, "VAR2 Name"="Vg") -> ("Header array"=w768:string[], "Data array"=w766:dbl[][])  [unwired: 14 in]
        n260 = local write "Imax vs time"(w773) -> ()
        n261 = local write "Imin vs time"(w770) -> ()
        n262 = local write "Ion vs time"(w723) -> ()
        n263 = local write "Ioff vs time"(w724) -> ()
        n264 = call "4155C Config Chart Colours.vi"("Numeric"=w719, "XY Graph 2"=w754) -> ()  [unwired: 6 in]
        n265 = call "4155C Config Chart Colours.vi"("Numeric"=w719, "XY Graph 2"=w753) -> ()  [unwired: 6 in]
        n266 = call "4155C Config Chart Colours.vi"("Numeric"=w719, "XY Graph 2"=w722) -> ()  [unwired: 6 in]
        n267 = call "4155C Config Chart Colours.vi"("Numeric"=w719, "XY Graph 2"=w721) -> ()  [unwired: 6 in]
        n268 = call "4155C Config Chart Colours.vi"("Numeric"=w719, "XY Graph 2"=w780) -> ()  [unwired: 6 in]
        n269 = call "4155C Write array to file.vi"("Byte Stream File Refnum"=w767, "Header"=w768, "Data Array"=w766, "error in (no error)"=w765) -> ("dup refnum"=w764:refnum<file>, "error out"=w763:errorcluster)  [unwired: 1 in]
        n270 = Close File(refnum=w764, error in=w763) -> (error out=w824:errorcluster)  [unwired: 1 out]
      }
      frame "output-fpp" {
        n271 = Number To Decimal String(number=w851) -> (decimal integer string=w905:string)  [unwired: 1 in]
        n272 = Bundle By Name(cluster=w881, "Emergency Stop"=w908) -> (w918:T2)
        n273 = Delete From Array(array=w896, index=0 ("Index")) -> (deleted portion=w894:string, array with subset deleted=w893:string[])  [unwired: 1 in]
        n274 = VISA Write(VISA resource name=w872, write buffer=":PAGE:CHAN:MODE SWE;" ("write buffer (\"\")"), error in (no error)=w869) -> (VISA resource name out=w871:refnum<visa-resource-name>, error out=w870:errorcluster)  [unwired: 1 out]
        n275 = Concatenate Strings(w904, "-outputfpp-" ("Substring"), w905, w850, ".txt" ("Substring")) -> (w907:string)
        n276 = case shown="\"d\", Default" w894 {
          tunnel: [w919 w920] -> w892
          frame "s" {
            w919 = u16 0 items=["Single", "Double"] ("sweep mode")
          }
          frame "d", Default {
            w920 = u16 1 items=["Single", "Double"] ("sweep mode")
          }
        }
        n277 = Fract/Exp String To Number(string=w893) -> (number=w875:dbl[])  [unwired: 3 in, 1 out]
        n278 = String To Path(string=w907) -> (path=w903:path)
        n279 = Index Array(array=w875, index #1=0 ("Index")) -> (element #1=w891:dbl, element #2=w890:dbl, element #3=w889:dbl)  [unwired: 2 in]
        n280 = Delete From Array(array=w875, length=3 ("Length"), index=0 ("Index")) -> (array with subset deleted=w874:dbl[])  [unwired: 1 out]
        n281 = Bundle By Name(cluster=w883, "Gate Start"=w891, "Gate Stop"=w890, "Gate Step (linear only)"=w889, "Gate Compliance"=w901, "Range mode"=w867, "Range"=w866) -> (w917:T6)
        n282 = Index Array(array=w874, index #1=0 ("Index")) -> (element #1=w886:dbl, element #2=w885:dbl, element #3=w884:dbl)  [unwired: 2 in]
        n283 = call <vilib>:"compatOverwrite.vi"("overwrite (F)"=TRUE) -> ("overwrite?"=w855:T8)
        n284 = Bundle By Name(cluster=w882, "Drain Start"=w886, "Drain Stop"=w885, "Drain Step"=w884, "Drain Compliance"=w902, "Range mode"=w865, "Range"=w868) -> (w916:T7)
        n285 = call "4155C Output-FPP.vi"("VISA resource name in"=w871, "Gate"=w917, "Drain"=w916, "Timings"=w900, "error in (no error)"=w870, "sweep mode"=w892, "Panel controls"=w918) -> ("VD"=w860:dbl[], "Outparams"=w863:T9, "VISA Resource Name out"=w898:refnum<visa-resource-name>, "Vprobe2"=w859:dbl[], "ID"=w858:dbl[], "IG"=w857:dbl[], "Vprobe1"=w856:dbl[], "error out"=w899:errorcluster)  [unwired: 13 in]
        n286 = Unbundle By Name(w863) -> ("V2 Step"=w864:dbl, "V2 Start"=w862:dbl, "Number of points"=w861:i32)
        n287 = Open/Create/Replace File(file path (use dialog)=w903, error in=w899, operation (0:open)=w855) -> (refnum out=w913:refnum<file>, error out=w914:errorcluster)  [unwired: 3 in, 1 out]
        n288 = call "4155C Make Big 2d array FPP.vi"("1D Var1"=w860, "1d ID"=w858, "1d Vp2"=w859, "1d IG"=w857, "1d Vp1"=w856, "VAR2 START"=w862, "Number of VAR2 steps"=w861, "VAR2 STEP"=w864, "VAR1 Name"="Vd", "Decimal places in header"=i8 1, "VAR2 Name"="Vg") -> ("Header array"=w909:string[], "Data array"=w910:dbl[][])  [unwired: 15 in]
        n289 = call "4155C Write array to file.vi"("Byte Stream File Refnum"=w913, "Header"=w909, "Data Array"=w910, "error in (no error)"=w914) -> ("dup refnum"=w911:refnum<file>, "error out"=w912:errorcluster)  [unwired: 1 in]
        n290 = Close File(refnum=w911, error in=w912) -> (error out=w897:errorcluster)  [unwired: 1 out]
      }
      frame "itime" {
        n291 = Delete From Array(array=w923, index=1) -> (deleted portion=w922:string)  [unwired: 1 in, 1 out]
        n292 = Delete From Array(array=w923, index=0 ("Index")) -> (deleted portion=w952:string)  [unwired: 1 in, 1 out]
        n293 = Fract/Exp String To Number(string=w922) -> (number=w921:dbl)  [unwired: 3 in, 1 out]
        n294 = case shown="\"l\"" w952 {
          tunnel: w951 -> [w957 w959 w963]
          tunnel: [w956 w958 w962] -> w944
          tunnel: w921 -> [w954 _ w961]
          frame "s" {
            w955 = u32 0 items=["short  ", "medium  ", "long  "] ("integration time 2")
            n295 = Bundle By Name(cluster=w957, "integration time"=w955, "Short/Long integration time"=w954) -> (w956:T5)
          }
          frame "m", Default {
            w960 = u32 1 items=["short  ", "medium  ", "long  "] ("integration time 2")
            n296 = Bundle By Name(cluster=w959, "integration time"=w960) -> (w958:T5)
          }
          frame "l" {
            w964 = u32 2 items=["short  ", "medium  ", "long  "] ("integration time 2")
            n297 = Bundle By Name(cluster=w963, "integration time"=w964, "Short/Long integration time"=w961) -> (w962:T5)
          }
        }
      }
      frame "pulsed" {
        n298 = Delete From Array(array=w993, index=0 ("Index")) -> (deleted portion=w994:string, array with subset deleted=w981:string[])  [unwired: 1 in]
        n299 = case shown="\"on\", Default" w994 {
          tunnel: w992 -> [w1004 w1007]
          tunnel: [w1003 w1006] -> w985
          tunnel: w981 -> [w1001 _]
          frame "on", Default {
            w1002 = u16 1 items=["Continuous", "Pulsed"] ("sweep method")
            n300 = Fract/Exp String To Number(string=w1001) -> (number=w999:dbl[])  [unwired: 3 in, 1 out]
            n301 = Index Array(array=w999, index #1=0 ("Index")) -> (element #1=w998:dbl, element #2=w997:dbl, element #3=w996:dbl)  [unwired: 2 in]
            n302 = Bundle By Name(cluster=w1004, "sweep method"=w1002, "Pulse period"=w998, "Base voltage"=w997, "Pulse width"=w996) -> (w1003:T5)
          }
          frame "off" {
            w1005 = u16 0 items=["Continuous", "Pulsed"] ("sweep method")
            n303 = Bundle By Name(cluster=w1007, "sweep method"=w1005) -> (w1006:T5)
          }
        }
      }
      frame "gaterangemode" {
        n304 = Delete From Array(array=w1034, index=0 ("Index")) -> (deleted portion=w1035:string)  [unwired: 1 in, 1 out]
        n305 = case shown="\"f\"" w1035 {
          tunnel: [w1037 w1038 w1039] -> w1024
          frame "a", Default {
            w1037 = u16 0 items=["Auto", "Limited", "Fixed"] ("Gate Range\nmode 2")
          }
          frame "f" {
            w1038 = u16 2 items=["Auto", "Limited", "Fixed"] ("Gate Range\nmode 2")
          }
          frame "l" {
            w1039 = u16 1 items=["Auto", "Limited", "Fixed"] ("Gate Range\nmode 2")
          }
        }
      }
      frame "gaterange" {
        (unwired) u8 11 items=["10fA  ", "100fA  ", "1nA  ", "10nA", "100nA", "1uA", "10uA", "100uA", "1mA", "10mA", "100mA", "1A"] ("Gate Range 2")
        n306 = Delete From Array(array=w1073, index=0 ("Index")) -> (deleted portion=w1063:string)  [unwired: 1 in, 1 out]
        n307 = Scan Value(string=w1063, format string="") -> (value=w1061:dbl)  [unwired: 1 in, 1 out]
        n308 = Logarithm Base 10(1:w1061) -> (0:w1060:dbl)
        n309 = Round To Nearest(number=w1060) -> (nearest integer value=w1059:dbl)
        n310 = Add(x=w1059, y=11.0) -> (x+y=w1057:dbl)
        n311 = To Unsigned Byte Integer(number=w1057) -> (unsigned 8bit integer=w1056:u8)
      }
      frame "drainrange" {
        (unwired) u8 11 items=["10fA  ", "100fA  ", "1nA  ", "10nA", "100nA", "1uA", "10uA", "100uA", "1mA", "10mA", "100mA", "1A"] ("Gate Range 2")
        n312 = Delete From Array(array=w1108, index=0 ("Index")) -> (deleted portion=w1099:string)  [unwired: 1 in, 1 out]
        n313 = Scan Value(string=w1099, format string="") -> (value=w1097:dbl)  [unwired: 1 in, 1 out]
        n314 = Logarithm Base 10(1:w1097) -> (0:w1096:dbl)
        n315 = Round To Nearest(number=w1096) -> (nearest integer value=w1095:dbl)
        n316 = Add(x=w1095, y=11.0) -> (x+y=w1093:dbl)
        n317 = To Unsigned Byte Integer(number=w1093) -> (unsigned 8bit integer=w1092:u8)
      }
      frame "drainrangemode" {
        n318 = Delete From Array(array=w1136, index=0 ("Index")) -> (deleted portion=w1137:string)  [unwired: 1 in, 1 out]
        n319 = case shown="\"f\"" w1137 {
          tunnel: [w1139 w1140 w1141] -> w1126
          frame "a", Default {
            w1139 = u16 0 items=["Auto", "Limited", "Fixed"] ("Gate Range\nmode 2")
          }
          frame "f" {
            w1140 = u16 2 items=["Auto", "Limited", "Fixed"] ("Gate Range\nmode 2")
          }
          frame "l" {
            w1141 = u16 1 items=["Auto", "Limited", "Fixed"] ("Gate Range\nmode 2")
          }
        }
      }
      frame "Error", Default {
      }
      frame "logfile" {
        n320 = Number To Decimal String(number=w1184) -> (decimal integer string=w1219:string)  [unwired: 1 in]
        n321 = Concatenate Strings(w1218, "logfile" ("Substring"), w1219, w1182, ".txt" ("Substring")) -> (w1216:string)
        n322 = String To Path(string=w1216) -> (path=w1189:path)
        n323 = Unbundle(w1215) -> ("integration time"=w1214:u32, "Short/Long integration time"=w1213:dbl, "hold time (sec)"=w1212:dbl, "delay time (sec)"=w1211:dbl, "Step Time (0 disables)"=w1210:dbl, "sweep method"=w1209:u16, "Pulse period"=w1208:dbl, "Base voltage"=w1207:dbl, "Pulse width"=w1206:dbl)
        n324 = Build Array(w1214, w1213, w1212, w1211, w1210, w1209, w1208, w1207, w1206, w1200, w1201, w1202, w1203, w1204, w1205) -> (w1193:dbl[])
        n325 = Insert Into Array(array=dbl[][] [] ("Input Array"), new element=w1193) -> (w1192:dbl[][])  [unwired: 2 in]
        n326 = call <vilib>:"compatOverwrite.vi"("overwrite (F)"=TRUE) -> ("overwrite?"=w1187:T8)
        n327 = Open/Create/Replace File(file path (use dialog)=w1189, error in=w1191, operation (0:open)=w1187) -> (refnum out=w1197:refnum<file>, error out=w1196:errorcluster)  [unwired: 3 in, 1 out]
        n328 = call "4155C Write array to file.vi"("Byte Stream File Refnum"=w1197, "Header"=string[] ["Int Time", "Short/Long Itime", "Hold time", "Delay time", "Step time", "Sweep method", "Pulse period", "Base Voltage", "Pulse width", "Drain compliance", "Gate compliance", "Gate range mode", "Gate range", "S/D range mode", "S/D range"], "Data Array"=w1192, "error in (no error)"=w1196) -> ("dup refnum"=w1199:refnum<file>, "error out"=w1198:errorcluster)  [unwired: 1 in]
        n329 = Close File(refnum=w1199, error in=w1198) -> (error out=w1190:errorcluster)  [unwired: 1 out]
      }
      frame "sample" {
        n330 = Number To Decimal String(number=w1237) -> (decimal integer string=w1285:string)  [unwired: 1 in]
        n331 = Fract/Exp String To Number(string=w1282) -> (number=w1243:dbl[])  [unwired: 3 in, 1 out]
        n332 = Concatenate Strings(w1260, "-sample-" ("Substring"), w1285, w1235, ".txt" ("Substring")) -> (w1283:string)
        n333 = Index Array(array=w1243, index=0 ("Index")) -> (element=w1280:dbl)
        n334 = String To Path(string=w1283) -> (path=w1264:path)
        n335 = Index Array(array=w1243, index=2 ("Index")) -> (element=w1276:dbl)
        n336 = Index Array(array=w1243, index=3 ("Index")) -> (element=w1245:dbl)
        n337 = Index Array(array=w1243, index=4 ("Index")) -> (element=w1242:dbl)
        n338 = call "4155C Config Sampling Measurements.vi"("Sampling interval"=w1242, "Sample time"=w1245, "Display on/off"=TRUE, "Timings"=w1251, "Num Points"=w1276, "error in (no error)"=w1287, "Drain Compliance"=w1286, "Gate Compliance"=w1261, "VISA session"=w1288) -> ("error out"=w1289:errorcluster, "dup VISA resource name"=w1290:refnum<visa-resource-name>)  [unwired: 1 in]
        n339 = Index Array(array=w1243, index=1 ("Index")) -> (element=w1277:dbl)
        n340 = call "4155C Take Sample.vi"("Emergency Stop"=w1257, "error in (no error)"=w1289, "Vd"=w1277, "Vg"=w1280, "VISA resource name in"=w1290) -> ("error out"=w1255:errorcluster, "Id"=w1292:dbl[], "Ig"=w1266:dbl[], "VISA Resource Name out"=w1253:refnum<visa-resource-name>, "Is"=w1291:dbl[], "Time"=w1270:dbl[])  [unwired: 1 in]
        n341 = Insert Into Array(array=dbl[][] [] ("Input Array"), new element=w1270) -> (w1269:dbl[][])  [unwired: 2 in]
        n342 = Insert Into Array(array=w1269, new element=w1266) -> (w1268:dbl[][])  [unwired: 2 in]
        n343 = Insert Into Array(array=w1268, new element=w1292) -> (w1267:dbl[][])  [unwired: 2 in]
        n344 = VISA Write(VISA resource name=w1253, write buffer=":DISP ON" ("write buffer (\"\")"), error in (no error)=w1255) -> (VISA resource name out=w1252:refnum<visa-resource-name>, error out=w1254:errorcluster)  [unwired: 1 out]
        n345 = Insert Into Array(array=w1267, new element=w1291) -> (w1259:dbl[][])  [unwired: 2 in]
        n346 = Transpose 2D Array(2D array=w1259) -> (transposed array=w1258:dbl[][])
        n347 = call <vilib>:"compatOverwrite.vi"("overwrite (F)"=TRUE) -> ("overwrite?"=w1240:T8)
        n348 = Open/Create/Replace File(file path (use dialog)=w1264, error in=w1254, operation (0:open)=w1240) -> (refnum out=w1273:refnum<file>, error out=w1272:errorcluster)  [unwired: 3 in, 1 out]
        n349 = call "4155C Write array to file.vi"("Byte Stream File Refnum"=w1273, "Header"=string[] ["Time /s", "Ig /A", "Id /A", "Is /A"], "Data Array"=w1258, "error in (no error)"=w1272) -> ("dup refnum"=w1275:refnum<file>, "error out"=w1274:errorcluster)  [unwired: 1 in]
        n350 = Close File(refnum=w1275, error in=w1274) -> (error out=w1262:errorcluster)  [unwired: 1 out]
      }
      frame "samplei" {
        n351 = Number To Decimal String(number=w1309) -> (decimal integer string=w1360:string)  [unwired: 1 in]
        n352 = Concatenate Strings(w1339, "-samplei-" ("Substring"), w1360, w1308, ".txt" ("Substring")) -> (w1358:string)
        n353 = Fract/Exp String To Number(string=w1357) -> (number=w1324:dbl[])  [unwired: 3 in, 1 out]
        n354 = String To Path(string=w1358) -> (path=w1342:path)
        n355 = Index Array(array=w1324, index=4 ("Index")) -> (element=w1318:dbl)
        n356 = Index Array(array=w1324, index=3 ("Index")) -> (element=w1319:dbl)
        n357 = Index Array(array=w1324, index=1 ("Index")) -> (element=w1321:dbl)
        n358 = Index Array(array=w1324, index=0 ("Index")) -> (element=w1322:dbl)
        n359 = Index Array(array=w1324, index=2 ("Index")) -> (element=w1320:dbl)
        n360 = call "4155C Config SamplingI Measurements.vi"("Sample time"=w1320, "Display on/off"=TRUE, "Timings"=w1331, "Num Points"=w1321, "error in (no error)"=w1362, "Sampling interval"=w1319, "VISA session"=w1363) -> ("error out"=w1364:errorcluster, "dup VISA resource name"=w1365:refnum<visa-resource-name>)  [unwired: 3 in]
        n361 = call "4155C Take SampleI.vi"("Emergency Stop"=w1336, "error in (no error)"=w1364, "Idg 2"=w1322, "Vdg compliance 2"=w1318, "VISA resource name in"=w1365) -> ("error out"=w1334:errorcluster, "Idg"=w1367:dbl[], "Vdg"=w1344:dbl[], "VISA Resource Name out"=w1332:refnum<visa-resource-name>, "Is"=w1366:dbl[], "Time"=w1348:dbl[])  [unwired: 1 in]
        n362 = Insert Into Array(array=dbl[][] [] ("Input Array"), new element=w1348) -> (w1347:dbl[][])  [unwired: 2 in]
        n363 = Insert Into Array(array=w1347, new element=w1344) -> (w1346:dbl[][])  [unwired: 2 in]
        n364 = Insert Into Array(array=w1346, new element=w1367) -> (w1345:dbl[][])  [unwired: 2 in]
        n365 = VISA Write(VISA resource name=w1332, write buffer=":DISP ON" ("write buffer (\"\")"), error in (no error)=w1334) -> (VISA resource name out=w1317:refnum<visa-resource-name>, error out=w1333:errorcluster)  [unwired: 1 out]
        n366 = Insert Into Array(array=w1345, new element=w1366) -> (w1338:dbl[][])  [unwired: 2 in]
        n367 = call <vilib>:"compatOverwrite.vi"("overwrite (F)"=TRUE) -> ("overwrite?"=w1312:T8)
        n368 = Open/Create/Replace File(file path (use dialog)=w1342, error in=w1333, operation (0:open)=w1312) -> (refnum out=w1351:refnum<file>, error out=w1350:errorcluster)  [unwired: 3 in, 1 out]
        n369 = Transpose 2D Array(2D array=w1338) -> (transposed array=w1337:dbl[][])
        n370 = call "4155C Write array to file.vi"("Byte Stream File Refnum"=w1351, "Header"=string[] ["Time /s", "Vdg /V", "Idg /A", "Is /A"], "Data Array"=w1337, "error in (no error)"=w1350) -> ("dup refnum"=w1353:refnum<file>, "error out"=w1352:errorcluster)  [unwired: 1 in]
        n371 = Close File(refnum=w1353, error in=w1352) -> (error out=w1315:errorcluster)  [unwired: 1 out]
        n372 = VISA Write(VISA resource name=w1317, write buffer=";:PAGE:SCON:STAN OFF;:PAGE:CHAN:VSU2:DIS;" ("write buffer (\"\")"), error in (no error)=w1315) -> (VISA resource name out=w1313:refnum<visa-resource-name>, error out=w1314:errorcluster)  [unwired: 1 out]
      }
      frame "#" {
        n373 = VISA Write(VISA resource name=w1388, write buffer=":DISP ON" ("write buffer (\"\")"), error in (no error)=w1387) -> (VISA resource name out=w1386:refnum<visa-resource-name>, error out=w1385:errorcluster)  [unwired: 1 out]
      }
      frame "stressV" {
        n374 = Number To Decimal String(number=w1412) -> (decimal integer string=w1453:string)  [unwired: 1 in]
        n375 = Concatenate Strings(w1437, "-stressV-" ("Substring"), w1453, w1411, ".txt" ("Substring")) -> (w1451:string)
        n376 = Fract/Exp String To Number(string=w1450) -> (number=w1423:dbl[])  [unwired: 3 in, 1 out]
        n377 = String To Path(string=w1451) -> (path=w1441:path)
        n378 = Index Array(array=w1423, index=3 ("Index")) -> (element=w1420:dbl)
        n379 = Index Array(array=w1423, index=1 ("Index")) -> (element=w1418:dbl)
        n380 = Index Array(array=w1423, index=0 ("Index")) -> (element=w1417:dbl)
        n381 = Index Array(array=w1423, index=4 ("Index")) -> (element=w1422:dbl)
        n382 = Index Array(array=w1423, index=2 ("Index")) -> (element=w1419:dbl)
        n383 = call "4155C Config V Stress.vi"("VISA session"=w1456, "ID compliance"=w1420, "VD"=w1418, "VG"=w1417, "IG compliance"=w1419, "error in (no error)"=w1455, "Display on/off"=TRUE) -> ("dup VISA resource name"=w1458:refnum<visa-resource-name>, "error out"=w1457:errorcluster)
        n384 = call "4155C Apply Stress.vi"("error in (no error)"=w1457, "Duration"=w1422, "Emergency Stop"=w1436, "VISA resource name in"=w1458) -> ("error out"=w1434:errorcluster, "VISA Resource Name out"=w1432:refnum<visa-resource-name>)
        n385 = VISA Write(VISA resource name=w1432, write buffer=":DISP ON" ("write buffer (\"\")"), error in (no error)=w1434) -> (VISA resource name out=w1431:refnum<visa-resource-name>, error out=w1433:errorcluster)  [unwired: 1 out]
        n386 = call <vilib>:"compatOverwrite.vi"("overwrite (F)"=TRUE) -> ("overwrite?"=w1416:T8)
        n387 = Open/Create/Replace File(file path (use dialog)=w1441, error in=w1433, operation (0:open)=w1416) -> (refnum out=w1444:refnum<file>, error out=w1443:errorcluster)  [unwired: 3 in, 1 out]
        n388 = call "4155C Write array to file.vi"("Byte Stream File Refnum"=w1444, "Header"=string[] ["V stress completed successfully", ""], "error in (no error)"=w1443) -> ("dup refnum"=w1446:refnum<file>, "error out"=w1445:errorcluster)  [unwired: 2 in]
        n389 = Close File(refnum=w1446, error in=w1445) -> (error out=w1439:errorcluster)  [unwired: 1 out]
      }
      frame "stressI" {
        n390 = Number To Decimal String(number=w1474) -> (decimal integer string=w1511:string)  [unwired: 1 in]
        n391 = Concatenate Strings(w1495, "-stressI-" ("Substring"), w1511, w1473, ".txt" ("Substring")) -> (w1509:string)
        n392 = Fract/Exp String To Number(string=w1508) -> (number=w1483:dbl[])  [unwired: 3 in, 1 out]
        n393 = Index Array(array=w1483, index=1 ("Index")) -> (element=w1479:dbl)
        n394 = Index Array(array=w1483, index=0 ("Index")) -> (element=w1480:dbl)
        n395 = call "4155C Config I Stress.vi"("VISA session"=w1514, "IDG"=w1480, "VDG compliance"=w1479, "error in (no error)"=w1513, "Display on/off"=TRUE) -> ("dup VISA resource name"=w1516:refnum<visa-resource-name>, "error out"=w1515:errorcluster)
        n396 = Index Array(array=w1483, index=2 ("Index")) -> (element=w1481:dbl)
        n397 = String To Path(string=w1509) -> (path=w1499:path)
        n398 = call "4155C Apply Stress.vi"("error in (no error)"=w1515, "Duration"=w1481, "Emergency Stop"=w1494, "VISA resource name in"=w1516) -> ("error out"=w1492:errorcluster, "VISA Resource Name out"=w1490:refnum<visa-resource-name>)
        n399 = VISA Write(VISA resource name=w1490, write buffer=":DISP ON" ("write buffer (\"\")"), error in (no error)=w1492) -> (VISA resource name out=w1489:refnum<visa-resource-name>, error out=w1491:errorcluster)  [unwired: 1 out]
        n400 = call <vilib>:"compatOverwrite.vi"("overwrite (F)"=TRUE) -> ("overwrite?"=w1478:T8)
        n401 = Open/Create/Replace File(file path (use dialog)=w1499, error in=w1491, operation (0:open)=w1478) -> (refnum out=w1502:refnum<file>, error out=w1501:errorcluster)  [unwired: 3 in, 1 out]
        n402 = call "4155C Write array to file.vi"("Byte Stream File Refnum"=w1502, "Header"=string[] ["I stress completed successfully", ""], "error in (no error)"=w1501) -> ("dup refnum"=w1504:refnum<file>, "error out"=w1503:errorcluster)  [unwired: 2 in]
        n403 = Close File(refnum=w1504, error in=w1503) -> (error out=w1497:errorcluster)  [unwired: 1 out]
      }
      frame "vsu2pulse" {
        n404 = Number To Decimal String(number=w1532) -> (decimal integer string=w1567:string)  [unwired: 1 in]
        n405 = Concatenate Strings(w1552, "-vsu2-" ("Substring"), w1567, w1531, ".txt" ("Substring")) -> (w1565:string)
        n406 = Fract/Exp String To Number(string=w1564) -> (number=w1540:dbl[])  [unwired: 3 in, 1 out]
        n407 = String To Path(string=w1565) -> (path=w1556:path)
        n408 = Index Array(array=w1540, index=1 ("Index")) -> (element=w1539:dbl)
        n409 = Index Array(array=w1540, index=0 ("Index")) -> (element=w1537:dbl)
        n410 = call "4155C Config VSU2 Stress.vi"("error in (no error)"=w1569, "VSU2"=w1537, "Display on/off"=TRUE, "VISA session"=w1570) -> ("error out"=w1571:errorcluster, "dup VISA resource name"=w1572:refnum<visa-resource-name>)
        n411 = call "4155C Apply Stress.vi"("error in (no error)"=w1571, "Duration"=w1539, "Emergency Stop"=w1551, "VISA resource name in"=w1572) -> ("error out"=w1549:errorcluster, "VISA Resource Name out"=w1547:refnum<visa-resource-name>)
        n412 = VISA Write(VISA resource name=w1547, write buffer=":DISP ON" ("write buffer (\"\")"), error in (no error)=w1549) -> (VISA resource name out=w1546:refnum<visa-resource-name>, error out=w1548:errorcluster)  [unwired: 1 out]
        n413 = call <vilib>:"compatOverwrite.vi"("overwrite (F)"=TRUE) -> ("overwrite?"=w1536:T8)
        n414 = Open/Create/Replace File(file path (use dialog)=w1556, error in=w1548, operation (0:open)=w1536) -> (refnum out=w1559:refnum<file>, error out=w1558:errorcluster)  [unwired: 3 in, 1 out]
        n415 = call "4155C Write array to file.vi"("Byte Stream File Refnum"=w1559, "Header"=string[] ["VSU2 pulse completed successfully", ""], "error in (no error)"=w1558) -> ("dup refnum"=w1561:refnum<file>, "error out"=w1560:errorcluster)  [unwired: 2 in]
        n416 = Close File(refnum=w1561, error in=w1560) -> (error out=w1554:errorcluster)  [unwired: 1 out]
      }
      frame "sample-fpp" {
        w1599 = string[] ["Time /s", "Id VgVd /A", "Ig VgVd /A", "Vp1 VgVd /V", "Vp2 VgVd /V"] ("Header")
        w1603 = "%d" ("format string")
        n417 = Number To Decimal String(number=w1588) -> (decimal integer string=w1651:string)  [unwired: 1 in]
        n418 = Fract/Exp String To Number(string=w1648) -> (number=w1636:dbl[])  [unwired: 3 in, 1 out]
        n419 = Concatenate Strings(w1642, "-samplefpp-" ("Substring"), w1651, w1587, ".txt" ("Substring")) -> (w1649:string)
        n420 = String To Path(string=w1649) -> (path=w1611:path)
        n421 = Index Array(array=w1636, index=0 ("Index")) -> (element=w1597:dbl)
        n422 = Index Array(array=w1636, index=1 ("Index")) -> (element=w1596:dbl)
        n423 = Index Array(array=w1636, index=2 ("Index")) -> (element=w1644:dbl)
        n424 = Index Array(array=w1636, index=3 ("Index")) -> (element=w1634:dbl)
        n425 = call "4155C Config Sampling Measurements FPP.vi"("VISA session"=w1654, "Num Points"=w1644, "Vg"=w1597, "Display on/off"=TRUE, "Gate Compliance"=w1643, "Drain Compliance"=w1652, "Standby"="Standby", "error in (no error)"=w1653, "Timings"=w1641, "Vd"=w1596, "Sample time"=w1634) -> ("dup VISA resource name"=w1613:refnum<visa-resource-name>, "error out"=w1612:errorcluster)  [unwired: 3 in]
        n426 = Number To Decimal String(number=w1597) -> (decimal integer string=w1623:string)  [unwired: 1 in]
        n427 = call "4155C Take Sample FPP.vi"("VISA resource name in"=w1613, "error in (no error)"=w1612, "Emergency Stop"=w1614) -> ("Time"=w1618:dbl[], "Vp1"=w1628:dbl[], "VISA Resource Name out"=w1594:refnum<visa-resource-name>, "Ig"=w1616:dbl[], "Id"=w1617:dbl[], "Vp2"=w1626:dbl[], "error out"=w1615:errorcluster)  [unwired: 10 in]
        n428 = Insert Into Array(array=dbl[][] [] ("Input Array"), new element=w1618) -> (w1632:dbl[][])  [unwired: 2 in]
        n429 = Number To Decimal String(number=w1596) -> (decimal integer string=w1621:string)  [unwired: 1 in]
        n430 = Insert Into Array(array=w1632, new element=w1617) -> (w1631:dbl[][])  [unwired: 2 in]
        n431 = Concatenate Strings("(Vg = " ("Substring"), w1623, "V, Vd = " ("Substring"), w1621, "V)" ("Substring")) -> (w1619:string)
        n432 = Insert Into Array(array=w1631, new element=w1616) -> (w1630:dbl[][])  [unwired: 2 in]
        n433 = Insert Into Array(array=w1630, new element=w1628) -> (w1627:dbl[][])  [unwired: 2 in]
        n434 = Insert Into Array(array=w1627, new element=w1626) -> (w1595:dbl[][])  [unwired: 2 in]
        n435 = Transpose 2D Array(2D array=w1595) -> (transposed array=w1625:dbl[][])
        n436 = call <vilib>:"compatOverwrite.vi"("overwrite (F)"=TRUE) -> ("overwrite?"=w1592:T8)
        n437 = Open/Create/Replace File(file path (use dialog)=w1611, error in=w1615, operation (0:open)=w1592) -> (refnum out=w1608:refnum<file>, error out=w1609:errorcluster)  [unwired: 3 in, 1 out]
        n438 = Array To Spreadsheet String(array=w1599, 3:w1603) -> (spreadsheet string=w1605:string)  [unwired: 1 in]
        n439 = Search and Replace String(replace all?=TRUE ("replace all? (F)"), input string=w1605, search string="VgVd", replace string=w1619) -> (result string=w1601:string)  [unwired: 4 in, 3 out]
        n440 = Spreadsheet String To Array(format string=w1603, spreadsheet string=w1601, array type (2D Dbl)=w1599) -> (array=w1600:string[])  [unwired: 1 in]
        n441 = call "4155C Write array to file.vi"("Byte Stream File Refnum"=w1608, "Header"=w1600, "Data Array"=w1625, "error in (no error)"=w1609) -> ("dup refnum"=w1606:refnum<file>, "error out"=w1607:errorcluster)  [unwired: 1 in]
        n442 = Close File(refnum=w1606, error in=w1607) -> (error out=w1593:errorcluster)  [unwired: 1 out]
      }
      frame "resample-fpp" {
        w1683 = string[] ["Time /s", "Id VgVd /A", "Ig VgVd /A", "Vp1 VgVd /V", "Vp2 VgVd /V"] ("Header")
        w1687 = "%d" ("format string")
        n443 = Number To Decimal String(number=w1669) -> (decimal integer string=w1727:string)  [unwired: 1 in]
        n444 = Fract/Exp String To Number(string=w1724) -> (number=w1676:dbl[])  [unwired: 3 in, 1 out]
        n445 = Concatenate Strings(w1720, "-resamplefpp-" ("Substring"), w1727, w1670, ".txt" ("Substring")) -> (w1725:string)
        n446 = String To Path(string=w1725) -> (path=w1695:path)
        n447 = Index Array(array=w1676, index=0 ("Index")) -> (element=w1682:dbl)
        n448 = Index Array(array=w1676, index=1 ("Index")) -> (element=w1681:dbl)
        n449 = Number To Decimal String(number=w1682) -> (decimal integer string=w1705:string)  [unwired: 1 in]
        n450 = call "4155C Take Sample FPP.vi"("VISA resource name in"=w1678, "error in (no error)"=w1677, "Emergency Stop"=w1696) -> ("Time"=w1700:dbl[], "Vp1"=w1710:dbl[], "VISA Resource Name out"=w1680:refnum<visa-resource-name>, "Ig"=w1698:dbl[], "Id"=w1699:dbl[], "Vp2"=w1708:dbl[], "error out"=w1697:errorcluster)  [unwired: 10 in]
        n451 = Insert Into Array(array=dbl[][] [] ("Input Array"), new element=w1700) -> (w1714:dbl[][])  [unwired: 2 in]
        n452 = Number To Decimal String(number=w1681) -> (decimal integer string=w1703:string)  [unwired: 1 in]
        n453 = Insert Into Array(array=w1714, new element=w1699) -> (w1713:dbl[][])  [unwired: 2 in]
        n454 = Concatenate Strings("(Vg = " ("Substring"), w1705, "V, Vd = " ("Substring"), w1703, "V)" ("Substring")) -> (w1701:string)
        n455 = Insert Into Array(array=w1713, new element=w1698) -> (w1712:dbl[][])  [unwired: 2 in]
        n456 = Insert Into Array(array=w1712, new element=w1710) -> (w1709:dbl[][])  [unwired: 2 in]
        n457 = Insert Into Array(array=w1709, new element=w1708) -> (w1675:dbl[][])  [unwired: 2 in]
        n458 = call <vilib>:"compatOverwrite.vi"("overwrite (F)"=TRUE) -> ("overwrite?"=w1674:T8)
        n459 = Open/Create/Replace File(file path (use dialog)=w1695, error in=w1697, operation (0:open)=w1674) -> (refnum out=w1692:refnum<file>, error out=w1693:errorcluster)  [unwired: 3 in, 1 out]
        n460 = Array To Spreadsheet String(array=w1683, 3:w1687) -> (spreadsheet string=w1689:string)  [unwired: 1 in]
        n461 = Transpose 2D Array(2D array=w1675) -> (transposed array=w1707:dbl[][])
        n462 = Search and Replace String(replace all?=TRUE ("replace all? (F)"), input string=w1689, search string="VgVd", replace string=w1701) -> (result string=w1685:string)  [unwired: 4 in, 3 out]
        n463 = Spreadsheet String To Array(format string=w1687, spreadsheet string=w1685, array type (2D Dbl)=w1683) -> (array=w1684:string[])  [unwired: 1 in]
        n464 = call "4155C Write array to file.vi"("Byte Stream File Refnum"=w1692, "Header"=w1684, "Data Array"=w1707, "error in (no error)"=w1693) -> ("dup refnum"=w1690:refnum<file>, "error out"=w1691:errorcluster)  [unwired: 1 in]
        n465 = Close File(refnum=w1690, error in=w1691) -> (error out=w1679:errorcluster)  [unwired: 1 out]
      }
      frame "serial" {
        n466 = local read "Termination char\n(0xA = '\\n' = LF)\n(0xD = '\\r' = CR)"() -> (w1750:u8)
        n467 = local read "Enable Termination\nChar (T)"() -> (w1751:bool)
        n468 = Index Array(array=w1758, index=0 ("Index")) -> (element=w1757:string)
        n469 = local read "parity"() -> (w1741:u16)
        n470 = local read "Delay before read (ms)"() -> (w1752:u32)
        n471 = local read "byte count"() -> (w1749:u32)
        n472 = local read "Timeout (ms)"() -> (w1748:u32)
        n473 = local read "VISA resource name"() -> (w1745:refnum<visa-resource-name>)
        n474 = local read "baud rate"() -> (w1744:u32)
        n475 = local read "Serial End Mode for Reads"() -> (w1743:u16)
        n476 = local read "data bits"() -> (w1742:u16)
        n477 = local read "stop bits"() -> (w1747:u16)
        n478 = local read "flow control"() -> (w1746:u16)
        n479 = call "Serial write and read v0.5.vi"("Delay before read (ms)"=w1752, "Termination char\n(0xA = '\\n' = LF)\n(0xD = '\\r' = CR)"=w1750, "Enable Termination\nChar (T)"=w1751, "parity"=w1741, "stop bits"=w1747, "string to write"=w1757, "flow control"=w1746, "byte count"=w1749, "Serial Settings:Serial End Mode for Reads"=w1743, "Timeout (ms)"=w1748, "error in (no error)"=w1763, "VISA resource name"=w1745, "baud rate"=w1744, "data bits"=w1742) -> ("Serial port output"=w1753:string, "error out"=w1762:errorcluster)
        n480 = Build Array (concatenate)(w1753, w1754) -> (w1755:string[])
      }
    }
    n481 = local read "Time Units"() -> (w62:u16)
    n482 = case shown="0" w62 {
      tunnel: ["Time (Seconds)" ("element") "Time (Minutes)" ("element") "Time (Hours)" ("element")] -> w102
      frame 0 {
      }
      frame 1, Default {
      }
      frame 2 {
      }
    }
    n483 = Build Array(w115, w70, w80, w79, w78, w77, w76, w75, w74, w73, w72, w71, w69) -> (w139:dbl[][])
    n484 = Transpose 2D Array(2D array=w139) -> (transposed array=w138:dbl[][])
    n485 = Concatenate Strings(w67, "-Imax_Imin_Ion_Ioff_vs_time.txt" ("Suffix (Imax,Imin,Ion,Ioff)")) -> (w149:string)
    n486 = Build Array(w102, "Is max (A)" ("VAR2 Name"), "Is min (A)" ("VAR2 Name"), "Id max (A)" ("VAR2 Name"), "Id min (A)" ("VAR2 Name"), "Ig max (A)" ("VAR2 Name"), "Ig min (A)" ("VAR2 Name"), "Is on (A)" ("VAR2 Name"), "Is off (A)" ("VAR2 Name"), "Id on (A)" ("VAR2 Name"), "Id off (A)" ("VAR2 Name"), "Ig on (A)" ("VAR2 Name"), "Ig off (A)" ("VAR2 Name")) -> (w144:string[])
    n487 = Array To Spreadsheet String(array=w138, 3:"%e" ("format string")) -> (spreadsheet string=w142:string)  [unwired: 1 in]
    n488 = Array To Spreadsheet String(array=w144, 3:"" ("format string")) -> (spreadsheet string=w143:string)  [unwired: 1 in]
    n489 = String To Path(string=w149) -> (path=w148:path)
    n490 = Build Array(w143, w142) -> (w141:string[])
    n491 = Write to Text File(file (use dialog)=w148, text=w141, error in=w113) -> (refnum out=w150:refnum<file>, error out=w140:errorcluster)  [unwired: 1 in, 1 out]
    n492 = Close File(refnum=w150, error in=w140) -> (error out=w66:errorcluster)  [unwired: 1 out]
    n493 = Concatenate Strings(w67, "-serial_port_output.txt" ("Suffix (serial port log)")) -> (w119:string)
    n494 = String To Path(string=w119) -> (path=w118:path)
    n495 = Build Array(w102, "Serial port input" ("VAR2 Name"), "Serial port output: ") -> (w106:string[])
    n496 = Array To Spreadsheet String(array=w110, 3:"" ("format string")) -> (spreadsheet string=w103:string)  [unwired: 1 in]
    n497 = Array To Spreadsheet String(array=w106, 3:"" ("format string")) -> (spreadsheet string=w104:string)  [unwired: 1 in]
    n498 = Build Array(w104, w103) -> (w105:string[])
    n499 = Array To Spreadsheet String(array=w109, 3:"" ("format string")) -> (spreadsheet string=w124:string)  [unwired: 1 in]
    n500 = Write to Text File(file (use dialog)=w118, text=w105, error in=w66) -> (refnum out=w120:refnum<file>, error out=w121:errorcluster)  [unwired: 1 in, 1 out]
    n501 = Close File(refnum=w120, error in=w121) -> (error out=w64:errorcluster)  [unwired: 1 out]
    n502 = local write "Serial port data"(w124) -> ()
  }
  "error out" <- w24
  "Timings Indicator" <- w12
  "Is max" <- w6
  "Id max" <- w6
  "Ig max" <- w6
  "Imax vs time" <- w2
  "I vs Vg" <- w2
  "Imin vs time" <- w2
  "I vs Vd" <- w2
  "Serial port data" <- "" ("Serial port data")
  "Is min" <- w5
  "Id min" <- w5
  "Ig min" <- w5
  "Ion vs time" <- w2
  "Ioff vs time" <- w2
  "Is on" <- w4
  "Id on" <- w4
  "Ig on" <- w4
  "Is off" <- w3
  "Id off" <- w3
  "Ig off" <- w3
